vi "Main.vi"() -> ()   [LabVIEW 2010]
uses:
  <vilib>/Utility/config.llb/Read Key (Path).vi
  <vilib>/Utility/config.llb/Write Key (Path).vi
  DLL-s/MakeFullImmitationStepDLL/Release/MakeFullImmitationStepDLL.dll
  <vilib>/Utility/config.llb/NI_LVConfig.lvlib
panel:
  out "toChanger":T1(array[cluster])
  out "subpanel VI ref":refnum<vi>
  out "VP 2 GUI Msg Cluster Array":cluster{"Names":string[], "Codes":i32[]}
  out "selected path":path
  out "End Number":i32
  out "Project":string
  out "VP input vars":T2
  out "VP output vars":T3
  out "VM input vars":T2
  out "VM2SCM Msg Cluster Array":cluster{"Names":string[], "Codes":i32[]}
  out "VM INP from SCM Msg Cluster Array":cluster{"Names":string[], "Codes":i32[]}
  out "SCM2CA Msg Cluster Array":cluster{"Names":string[], "Codes":i32[]}
  out "SCM-SCM2VP Msg Cluster Array":cluster{"Names":string[], "Codes":i32[]}
  out "SCM2VM Msg Cluster Array":cluster{"Names":string[], "Codes":i32[]}
  out "VM2GUI Msg Cluster Array":cluster{"Names":string[], "Codes":i32[]}
  out "SCM STATES":string[][](array[string])
  out "SCM PROCESSES":string[](array[string])=["Инициализация", "ОстановВсехПроцессовИстартПроцИнициализация", "КонтрольДостоверности", "КонтрольДостоверностиОткрытияЗатвораВакуумного", "КонтрольДостоверностиОткрЗатВакуумного", "КонтрольДостоверностиЗакрЗатВакуумного", "КонтрольДостоверностиСостоянияСапуна", "КонтрольДостоверностиСостоянияУстройстваПлавПуска", "КонтрольДостоверностиСостоянияПитанияВакуумногоНасоса", "КонтрольДостоверностиСостоянияПитанияВентилятора", "КонтрольДостоверностиСостоянияПитанияРегТемпературы", "КонтрольДостоверностиСостоянияПитанияРегУровня", "КонтрольДостоверностиУровняВодыМинимум", "КонтрольДостоверностиУровняВодыМаксимум", "КонтрольДостоверностиСостоянияПитанияНасОхлаждения", "ЧтениеФактПараметров_с_Датчиков", "РЕГУЛЯТОР_ТРАФИКА", "ЧтениеКольцевогоБуфера", "ОбработкаКомандИзмененияНП_от_ГУИ", "ОбработкаКомандУправления_от_ГУИ", "КонтрольИзменения_ФП_P_ВбакеКомпрессора", "КонтрольИзменения_ФП_P_Впатрубке", "КонтрольИзменения_ФП_T_Врубашке", "КонтрольИзменения_ФП_T_Вбаке", "КонтрольИзменения_ФП_P_ВтрубеСидер", "КонтрольВеличиныОткачкиВауумнойТрубыСидеростата", "КонтрольГотовностиВакуума_в_Вакуумной_Трубе", "КонтрольУровняВодыБакаОхлаждения", "КонтрольТемпературыВодыБакаОхлаждения", "КонтрольТемпературыРубашкиОхлаждения", "КонтрольДавленияВбакеКомпрессора", "ВКЛ_ПИТ_ВЕНТИЛЯТОР", "ВЫК_ПИТ_ВЕНТИЛЯТОР", "КонтрольСостоянияПитанияВентилятора", "КонтрольСпонтанногоВыключенияВентилятора", "КонтрольСпонтанногоВключенияВентилятора", "КонтрольСостоянияЗатвораВакуумного", "ОТКР_ЗАТВОР_ВАК", "ЗАКР_ЗАТВОР_ВАК", "КонтрольСпонтанногоЗакрытияЗатвораВакуумного", "КонтрольСпонтанногоОткрытияЗатвораВакуумного", "ОТКР_САПУН", "ЗАКР_САПУН", "КонтрольСостоянияПитанияСапуна", "КонтрольСпонтанногоЗакрытияСапуна", "КонтрольСпонтанногоОткрытияСапуна", "ВКЛ_ПИТ_ВАК_НАСОСА", "ВЫК_ПИТ_ВАК_НАСОСА", "КонтрольСостоянияПитанияВакуумногоНасоса", "КонтрольСпонтанногоВыключенияВакНасоса", "КонтрольСпонтанногоВключенияВакНасоса", "ВКЛ_ПИТ_РЕГ_Т", "ВЫК_ПИТ_РЕГ_Т", "КонтрольСостоянияПитанияРЕГ_Т", "КонтрольСпонтанногоВыключенияРЕГ_Т", "КонтрольСпонтанногоВключенияРЕГ_Т", "ВКЛ_ПИТ_РЕГ_УР", "ВЫК_ПИТ_РЕГ_УР", "КонтрольСостоянияПитанияРЕГ_УР", "КонтрольСпонтанногоВыключенияРЕГ_УР", "КонтрольСпонтанногоВключенияРЕГ_УР", "ВКЛ_ПИТ_НАС_ОХЛ", "ВЫК_ПИТ_НАС_ОХЛ", "КонтрольСостоянияПитанияНАС_ОХЛ", "КонтрольСпонтанногоВыключенияНасосаОхлаждения", "КонтрольСпонтанногоВключенияНасосаОхлаждения", "ВКЛ_УСТР_ПЛАВ_ПУСКА", "ВЫК_УСТР_ПЛАВ_ПУСКА", "КонтрольСостоянияПитанияПЛАВ_ПУСКА", "КонтрольСпонтанногоВыключенияПлавнПуска", "КонтрольСпонтанногоВключенияПлавнПуска", "ВКЛ_ВАКУУМИРОВАНИЕ_ТРУБЫ", "ВЫК_ВАКУУМИРОВАНИЕ_ТРУБЫ", "ВКЛ_ВАКУУМНУЮ_ПОДСИСТЕМУ", "ВЫК_ВАКУУМНУЮ_ПОДСИСТЕМУ"]
  out "VM STATES":string[][](array[string])
  out "VM PROCESSES":string[](array[string])=["Инициализация", "ОстановВсехПроцессовИстартПроцИнициализация", "КонтрольДостоверности", "КонтрольДостоверностиОткрытияЗатвораВакуумного", "КонтрольДостоверностиОткрЗатВакуумного", "КонтрольДостоверностиЗакрЗатВакуумного", "КонтрольДостоверностиСостоянияСапуна", "КонтрольДостоверностиСостоянияУстройстваПлавПуска", "КонтрольДостоверностиСостоянияПитанияВакуумногоНасоса", "КонтрольДостоверностиСостоянияПитанияВентилятора", "КонтрольДостоверностиСостоянияПитанияРегТемпературы", "КонтрольДостоверностиСостоянияПитанияРегУровня", "КонтрольДостоверностиУровняВодыМинимум", "КонтрольДостоверностиУровняВодыМаксимум", "КонтрольДостоверностиСостоянияПитанияНасОхлаждения", "ЧтениеФактПараметров_с_Датчиков", "РЕГУЛЯТОР_ТРАФИКА", "ЧтениеКольцевогоБуфера", "ОбработкаКомандИзмененияНП_от_ГУИ", "ОбработкаКомандУправления_от_ГУИ", "КонтрольИзменения_ФП_P_ВбакеКомпрессора", "КонтрольИзменения_ФП_P_Впатрубке", "КонтрольИзменения_ФП_T_Врубашке", "КонтрольИзменения_ФП_T_Вбаке", "КонтрольИзменения_ФП_P_ВтрубеСидер", "КонтрольВеличиныОткачкиВауумнойТрубыСидеростата", "КонтрольГотовностиВакуума_в_Вакуумной_Трубе", "КонтрольУровняВодыБакаОхлаждения", "КонтрольТемпературыВодыБакаОхлаждения", "КонтрольТемпературыРубашкиОхлаждения", "КонтрольДавленияВбакеКомпрессора", "ВКЛ_ПИТ_ВЕНТИЛЯТОР", "ВЫК_ПИТ_ВЕНТИЛЯТОР", "КонтрольСостоянияПитанияВентилятора", "КонтрольСпонтанногоВыключенияВентилятора", "КонтрольСпонтанногоВключенияВентилятора", "КонтрольСостоянияЗатвораВакуумного", "ОТКР_ЗАТВОР_ВАК", "ЗАКР_ЗАТВОР_ВАК", "КонтрольСпонтанногоЗакрытияЗатвораВакуумного", "КонтрольСпонтанногоОткрытияЗатвораВакуумного", "ОТКР_САПУН", "ЗАКР_САПУН", "КонтрольСостоянияПитанияСапуна", "КонтрольСпонтанногоЗакрытияСапуна", "КонтрольСпонтанногоОткрытияСапуна", "ВКЛ_ПИТ_ВАК_НАСОСА", "ВЫК_ПИТ_ВАК_НАСОСА", "КонтрольСостоянияПитанияВакуумногоНасоса", "КонтрольСпонтанногоВыключенияВакНасоса", "КонтрольСпонтанногоВключенияВакНасоса", "ВКЛ_ПИТ_РЕГ_Т", "ВЫК_ПИТ_РЕГ_Т", "КонтрольСостоянияПитанияРЕГ_Т", "КонтрольСпонтанногоВыключенияРЕГ_Т", "КонтрольСпонтанногоВключенияРЕГ_Т", "ВКЛ_ПИТ_РЕГ_УР", "ВЫК_ПИТ_РЕГ_УР", "КонтрольСостоянияПитанияРЕГ_УР", "КонтрольСпонтанногоВыключенияРЕГ_УР", "КонтрольСпонтанногоВключенияРЕГ_УР", "ВКЛ_ПИТ_НАС_ОХЛ", "ВЫК_ПИТ_НАС_ОХЛ", "КонтрольСостоянияПитанияНАС_ОХЛ", "КонтрольСпонтанногоВыключенияНасосаОхлаждения", "КонтрольСпонтанногоВключенияНасосаОхлаждения", "ВКЛ_УСТР_ПЛАВ_ПУСКА", "ВЫК_УСТР_ПЛАВ_ПУСКА", "КонтрольСостоянияПитанияПЛАВ_ПУСКА", "КонтрольСпонтанногоВыключенияПлавнПуска", "КонтрольСпонтанногоВключенияПлавнПуска", "ВКЛ_ВАКУУМИРОВАНИЕ_ТРУБЫ", "ВЫК_ВАКУУМИРОВАНИЕ_ТРУБЫ", "ВКЛ_ВАКУУМНУЮ_ПОДСИСТЕМУ", "ВЫК_ВАКУУМНУЮ_ПОДСИСТЕМУ"]
  out "VP STATES":string[][](array[string])
  out "VP PROCESSES":string[](array[string])=["Инициализация", "ОстановВсехПроцессовИстартПроцИнициализация", "КонтрольДостоверности", "КонтрольДостоверностиОткрытияЗатвораВакуумного", "КонтрольДостоверностиОткрЗатВакуумного", "КонтрольДостоверностиЗакрЗатВакуумного", "КонтрольДостоверностиСостоянияСапуна", "КонтрольДостоверностиСостоянияУстройстваПлавПуска", "КонтрольДостоверностиСостоянияПитанияВакуумногоНасоса", "КонтрольДостоверностиСостоянияПитанияВентилятора", "КонтрольДостоверностиСостоянияПитанияРегТемпературы", "КонтрольДостоверностиСостоянияПитанияРегУровня", "КонтрольДостоверностиУровняВодыМинимум", "КонтрольДостоверностиУровняВодыМаксимум", "КонтрольДостоверностиСостоянияПитанияНасОхлаждения", "ЧтениеФактПараметров_с_Датчиков", "РЕГУЛЯТОР_ТРАФИКА", "ЧтениеКольцевогоБуфера", "ОбработкаКомандИзмененияНП_от_ГУИ", "ОбработкаКомандУправления_от_ГУИ", "КонтрольИзменения_ФП_P_ВбакеКомпрессора", "КонтрольИзменения_ФП_P_Впатрубке", "КонтрольИзменения_ФП_T_Врубашке", "КонтрольИзменения_ФП_T_Вбаке", "КонтрольИзменения_ФП_P_ВтрубеСидер", "КонтрольВеличиныОткачкиВауумнойТрубыСидеростата", "КонтрольГотовностиВакуума_в_Вакуумной_Трубе", "КонтрольУровняВодыБакаОхлаждения", "КонтрольТемпературыВодыБакаОхлаждения", "КонтрольТемпературыРубашкиОхлаждения", "КонтрольДавленияВбакеКомпрессора", "ВКЛ_ПИТ_ВЕНТИЛЯТОР", "ВЫК_ПИТ_ВЕНТИЛЯТОР", "КонтрольСостоянияПитанияВентилятора", "КонтрольСпонтанногоВыключенияВентилятора", "КонтрольСпонтанногоВключенияВентилятора", "КонтрольСостоянияЗатвораВакуумного", "ОТКР_ЗАТВОР_ВАК", "ЗАКР_ЗАТВОР_ВАК", "КонтрольСпонтанногоЗакрытияЗатвораВакуумного", "КонтрольСпонтанногоОткрытияЗатвораВакуумного", "ОТКР_САПУН", "ЗАКР_САПУН", "КонтрольСостоянияПитанияСапуна", "КонтрольСпонтанногоЗакрытияСапуна", "КонтрольСпонтанногоОткрытияСапуна", "ВКЛ_ПИТ_ВАК_НАСОСА", "ВЫК_ПИТ_ВАК_НАСОСА", "КонтрольСостоянияПитанияВакуумногоНасоса", "КонтрольСпонтанногоВыключенияВакНасоса", "КонтрольСпонтанногоВключенияВакНасоса", "ВКЛ_ПИТ_РЕГ_Т", "ВЫК_ПИТ_РЕГ_Т", "КонтрольСостоянияПитанияРЕГ_Т", "КонтрольСпонтанногоВыключенияРЕГ_Т", "КонтрольСпонтанногоВключенияРЕГ_Т", "ВКЛ_ПИТ_РЕГ_УР", "ВЫК_ПИТ_РЕГ_УР", "КонтрольСостоянияПитанияРЕГ_УР", "КонтрольСпонтанногоВыключенияРЕГ_УР", "КонтрольСпонтанногоВключенияРЕГ_УР", "ВКЛ_ПИТ_НАС_ОХЛ", "ВЫК_ПИТ_НАС_ОХЛ", "КонтрольСостоянияПитанияНАС_ОХЛ", "КонтрольСпонтанногоВыключенияНасосаОхлаждения", "КонтрольСпонтанногоВключенияНасосаОхлаждения", "ВКЛ_УСТР_ПЛАВ_ПУСКА", "ВЫК_УСТР_ПЛАВ_ПУСКА", "КонтрольСостоянияПитанияПЛАВ_ПУСКА", "КонтрольСпонтанногоВыключенияПлавнПуска", "КонтрольСпонтанногоВключенияПлавнПуска", "ВКЛ_ВАКУУМИРОВАНИЕ_ТРУБЫ", "ВЫК_ВАКУУМИРОВАНИЕ_ТРУБЫ", "ВКЛ_ВАКУУМНУЮ_ПОДСИСТЕМУ", "ВЫК_ВАКУУМНУЮ_ПОДСИСТЕМУ"]
  out "VP Cluster":T4
  out "CA output vars":T3
  out "CA input vars":T2
  out "CA2GUI Msg Cluster Array":cluster{"Names":string[], "Codes":i32[]}
  out "COM2CA MSG Cluster Array":cluster{"Names":string[], "Codes":i32[]}
  out "CA STATES":string[][](array[string])
  out "CA PROCESSES":string[](array[string])=["Инициализация", "ОстановВсехПроцессовИстартПроцИнициализация", "КонтрольДостоверности", "КонтрольДостоверностиОткрытияЗатвораВакуумного", "КонтрольДостоверностиОткрЗатВакуумного", "КонтрольДостоверностиЗакрЗатВакуумного", "КонтрольДостоверностиСостоянияСапуна", "КонтрольДостоверностиСостоянияУстройстваПлавПуска", "КонтрольДостоверностиСостоянияПитанияВакуумногоНасоса", "КонтрольДостоверностиСостоянияПитанияВентилятора", "КонтрольДостоверностиСостоянияПитанияРегТемпературы", "КонтрольДостоверностиСостоянияПитанияРегУровня", "КонтрольДостоверностиУровняВодыМинимум", "КонтрольДостоверностиУровняВодыМаксимум", "КонтрольДостоверностиСостоянияПитанияНасОхлаждения", "ЧтениеФактПараметров_с_Датчиков", "РЕГУЛЯТОР_ТРАФИКА", "ЧтениеКольцевогоБуфера", "ОбработкаКомандИзмененияНП_от_ГУИ", "ОбработкаКомандУправления_от_ГУИ", "КонтрольИзменения_ФП_P_ВбакеКомпрессора", "КонтрольИзменения_ФП_P_Впатрубке", "КонтрольИзменения_ФП_T_Врубашке", "КонтрольИзменения_ФП_T_Вбаке", "КонтрольИзменения_ФП_P_ВтрубеСидер", "КонтрольВеличиныОткачкиВауумнойТрубыСидеростата", "КонтрольГотовностиВакуума_в_Вакуумной_Трубе", "КонтрольУровняВодыБакаОхлаждения", "КонтрольТемпературыВодыБакаОхлаждения", "КонтрольТемпературыРубашкиОхлаждения", "КонтрольДавленияВбакеКомпрессора", "ВКЛ_ПИТ_ВЕНТИЛЯТОР", "ВЫК_ПИТ_ВЕНТИЛЯТОР", "КонтрольСостоянияПитанияВентилятора", "КонтрольСпонтанногоВыключенияВентилятора", "КонтрольСпонтанногоВключенияВентилятора", "КонтрольСостоянияЗатвораВакуумного", "ОТКР_ЗАТВОР_ВАК", "ЗАКР_ЗАТВОР_ВАК", "КонтрольСпонтанногоЗакрытияЗатвораВакуумного", "КонтрольСпонтанногоОткрытияЗатвораВакуумного", "ОТКР_САПУН", "ЗАКР_САПУН", "КонтрольСостоянияПитанияСапуна", "КонтрольСпонтанногоЗакрытияСапуна", "КонтрольСпонтанногоОткрытияСапуна", "ВКЛ_ПИТ_ВАК_НАСОСА", "ВЫК_ПИТ_ВАК_НАСОСА", "КонтрольСостоянияПитанияВакуумногоНасоса", "КонтрольСпонтанногоВыключенияВакНасоса", "КонтрольСпонтанногоВключенияВакНасоса", "ВКЛ_ПИТ_РЕГ_Т", "ВЫК_ПИТ_РЕГ_Т", "КонтрольСостоянияПитанияРЕГ_Т", "КонтрольСпонтанногоВыключенияРЕГ_Т", "КонтрольСпонтанногоВключенияРЕГ_Т", "ВКЛ_ПИТ_РЕГ_УР", "ВЫК_ПИТ_РЕГ_УР", "КонтрольСостоянияПитанияРЕГ_УР", "КонтрольСпонтанногоВыключенияРЕГ_УР", "КонтрольСпонтанногоВключенияРЕГ_УР", "ВКЛ_ПИТ_НАС_ОХЛ", "ВЫК_ПИТ_НАС_ОХЛ", "КонтрольСостоянияПитанияНАС_ОХЛ", "КонтрольСпонтанногоВыключенияНасосаОхлаждения", "КонтрольСпонтанногоВключенияНасосаОхлаждения", "ВКЛ_УСТР_ПЛАВ_ПУСКА", "ВЫК_УСТР_ПЛАВ_ПУСКА", "КонтрольСостоянияПитанияПЛАВ_ПУСКА", "КонтрольСпонтанногоВыключенияПлавнПуска", "КонтрольСпонтанногоВключенияПлавнПуска", "ВКЛ_ВАКУУМИРОВАНИЕ_ТРУБЫ", "ВЫК_ВАКУУМИРОВАНИЕ_ТРУБЫ", "ВКЛ_ВАКУУМНУЮ_ПОДСИСТЕМУ", "ВЫК_ВАКУУМНУЮ_ПОДСИСТЕМУ"]
  out "CA DESCR":T5
  out "VM DESCR":T6
  out "exists":bool
  out "Scalar":bool
  in  "Проект":path
  out "Stop Ver Button":bool
  in  "Pause":bool
  out "Верификация запущена":bool
  out "error":i32
  in  "verifier2scenariousControlOutMsgs":cluster{"MSG":i16, "param":i32, "Type":i16}[](array[cluster])
  out "Verification":bool
  in  "scenarioStates":cluster{"TimeInState":u16, "cur_state":i8}[](array[cluster])
  in  "verStates":cluster{"TimeInState":u16, "cur_state":i8}[](array[cluster])
  in  "vplantStates":cluster{"TimeInState":u16, "cur_state":i8}[](array[cluster])
  in  "algStates":cluster{"TimeInState":u16, "cur_state":i8}[](array[cluster])
  in  "virtualPlant2GUIOutputMsgs":cluster{"MSG":i16, "param":i32, "Type":i16}[](array[cluster])
  in  "verifier2GUIOutputMsgs":cluster{"MSG":i16, "param":i32, "Type":i16}[](array[cluster])
  in  "algOutputMsgs":T7(array[cluster])
  in  "scenarios2VerifierOutputMsgs":cluster{"MSG":i16, "param":i32, "Type":i16}[](array[cluster])
  in  "scenarios2VirtPlantOutputMsgs":cluster{"MSG":i16, "param":i32, "Type":i16}[](array[cluster])
  in  "scenarios2AlgOutputMsgs":cluster{"MSG":i16, "param":i32, "Type":i16}[](array[cluster])
  in  "algOutputPorts":i8[](array[numeric])
  in  "algInputPorts":i8[](array[numeric])
  in  "TEST MODE":bool
  in  "Open editor":bool
  in  "START Button":bool
  out "VM vi reference":refnum<vi> caption="CA vi reference"
  out "SCB vi reference":refnum<vi> caption="CA vi reference"
  out "VP vi reference":refnum<vi> caption="CA vi reference"
  out "CA vi reference":refnum<vi>
  out "error out":errorcluster
  in  "Открыть панель БВ":bool
  in  "Открыть панель БУС":bool
  in  "Открыть панель АУ":bool
  in  "stop":bool
  in  "Открыть панель ВОУ":bool
  out "Автоматический режим работы":bool
  in  "Режим работы:":bool
  # "Ручной"
  # "Автоматический"
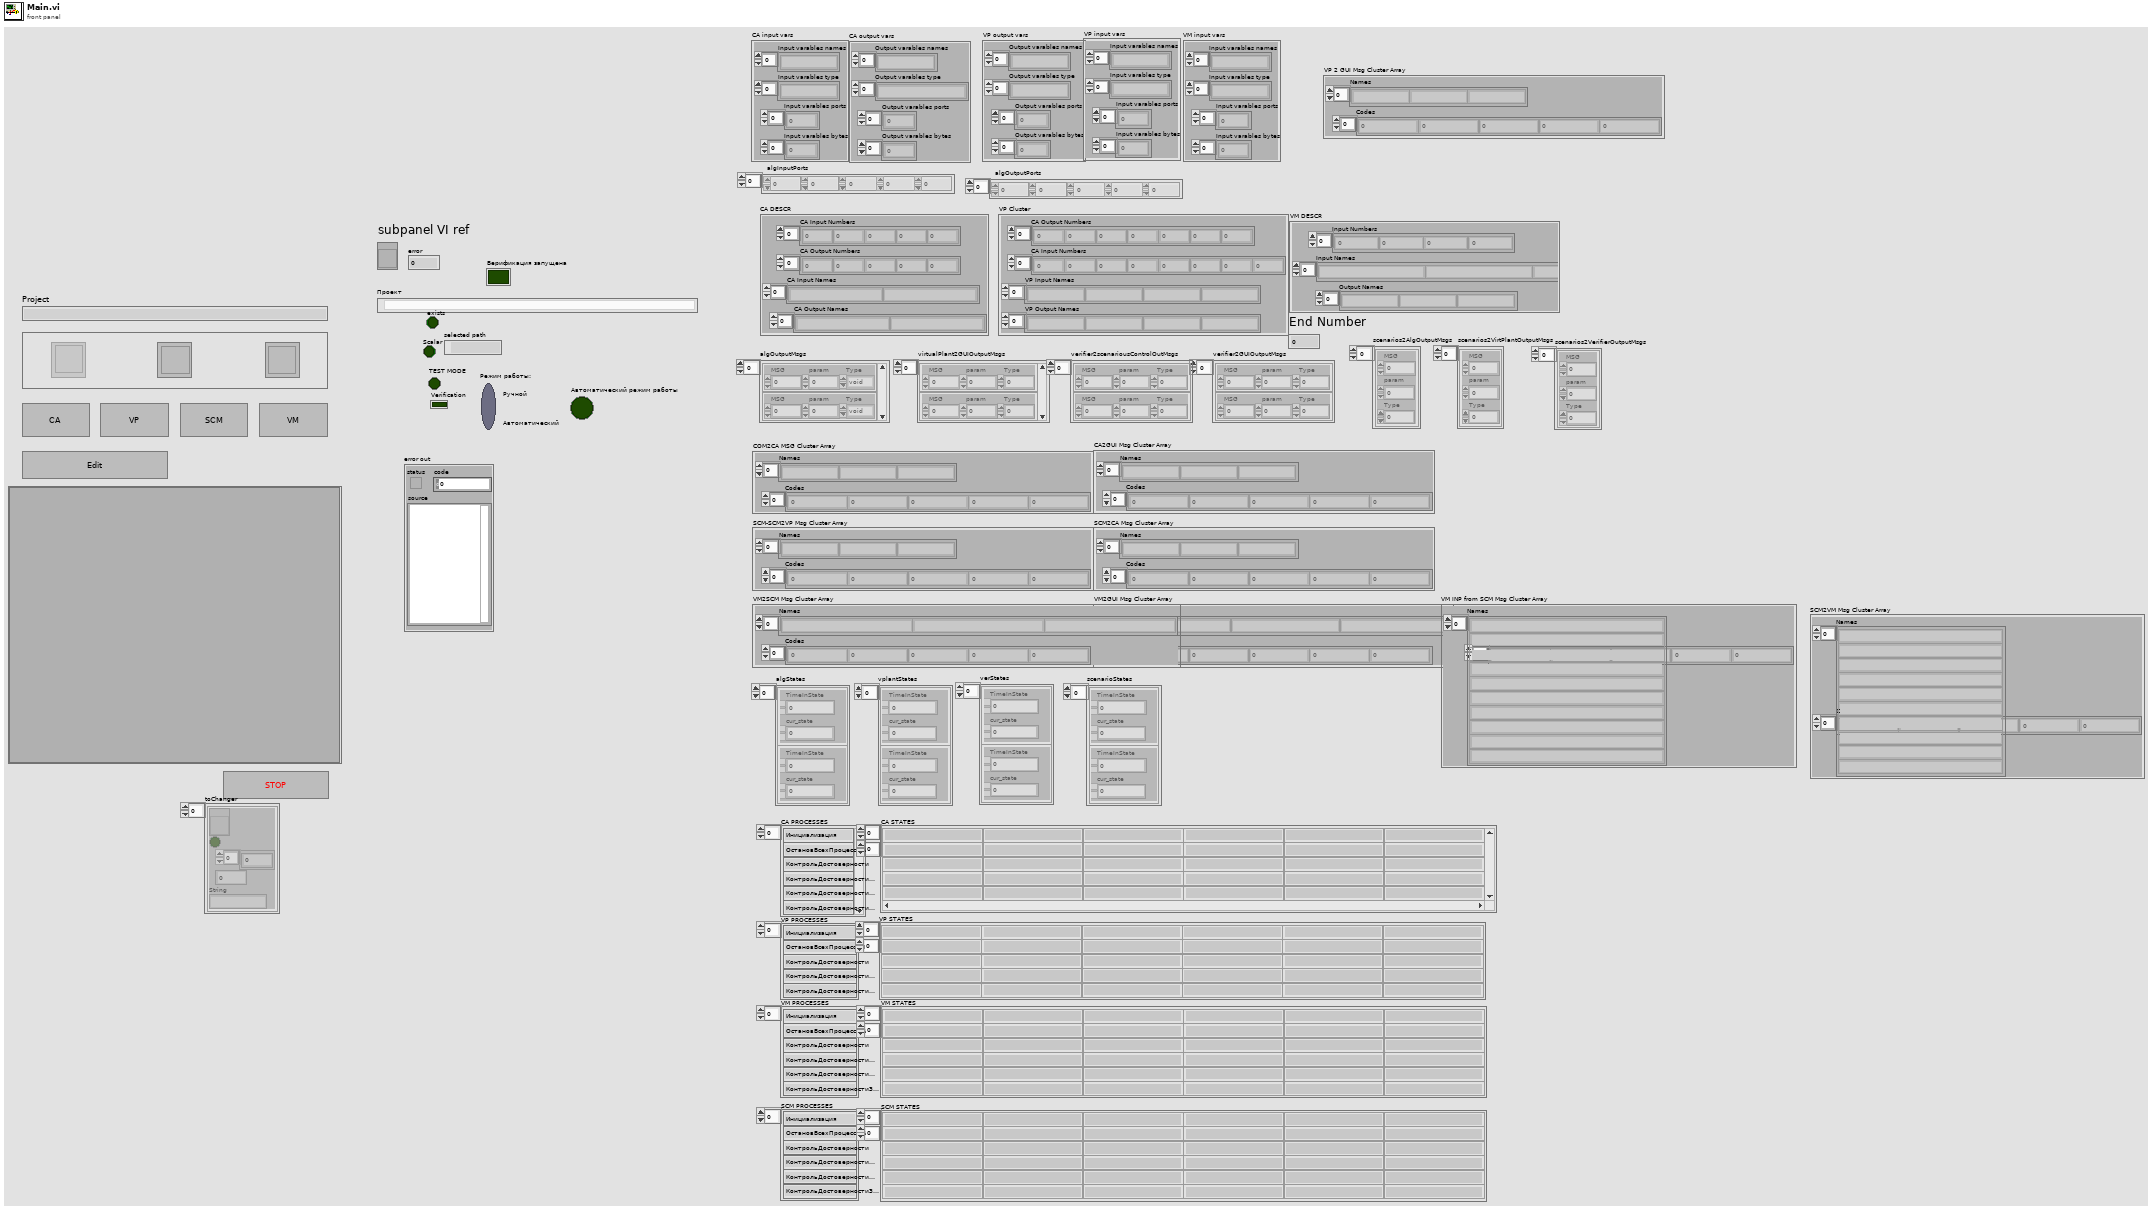
[diagram p1: front panel]
types:
  T1 = cluster{refnum<vi>, bool, i32[], i32, "String":string}[]
  T2 = cluster{"Input varables names":string[], "Input varables type":string[], "Input varables ports":i32[], "Input varables bytes":i32[]}
  T3 = cluster{"Output varables names":string[], "Output varables type":string[], "Output varables ports":i32[], "Output varables bytes":i32[]}
  T4 = cluster{"CA Output Numbers ":i32[], "CA Input Numbers":i32[], "VP Input Names":string[], "VP Output Names ":string[]}
  T5 = cluster{"CA Input Numbers":i32[], "CA Output Numbers ":i32[], "CA Input Names":string[], "CA Output Names ":string[]}
  T6 = cluster{"Input Numbers":i32[], "Input Names":string[], "Output Names ":string[]}
  T7 = cluster{"MSG":i16, "param":i32, "Type":enum16{"void", "byte", "int", "float"}}[]
  T8 = enum8{"Enabled", "Disabled", "Disabled and Grayed Out"}
  T9 = typedef "NI_LVConfig.lvlib/Config Data RefNum.ctl" = refnum<k1>
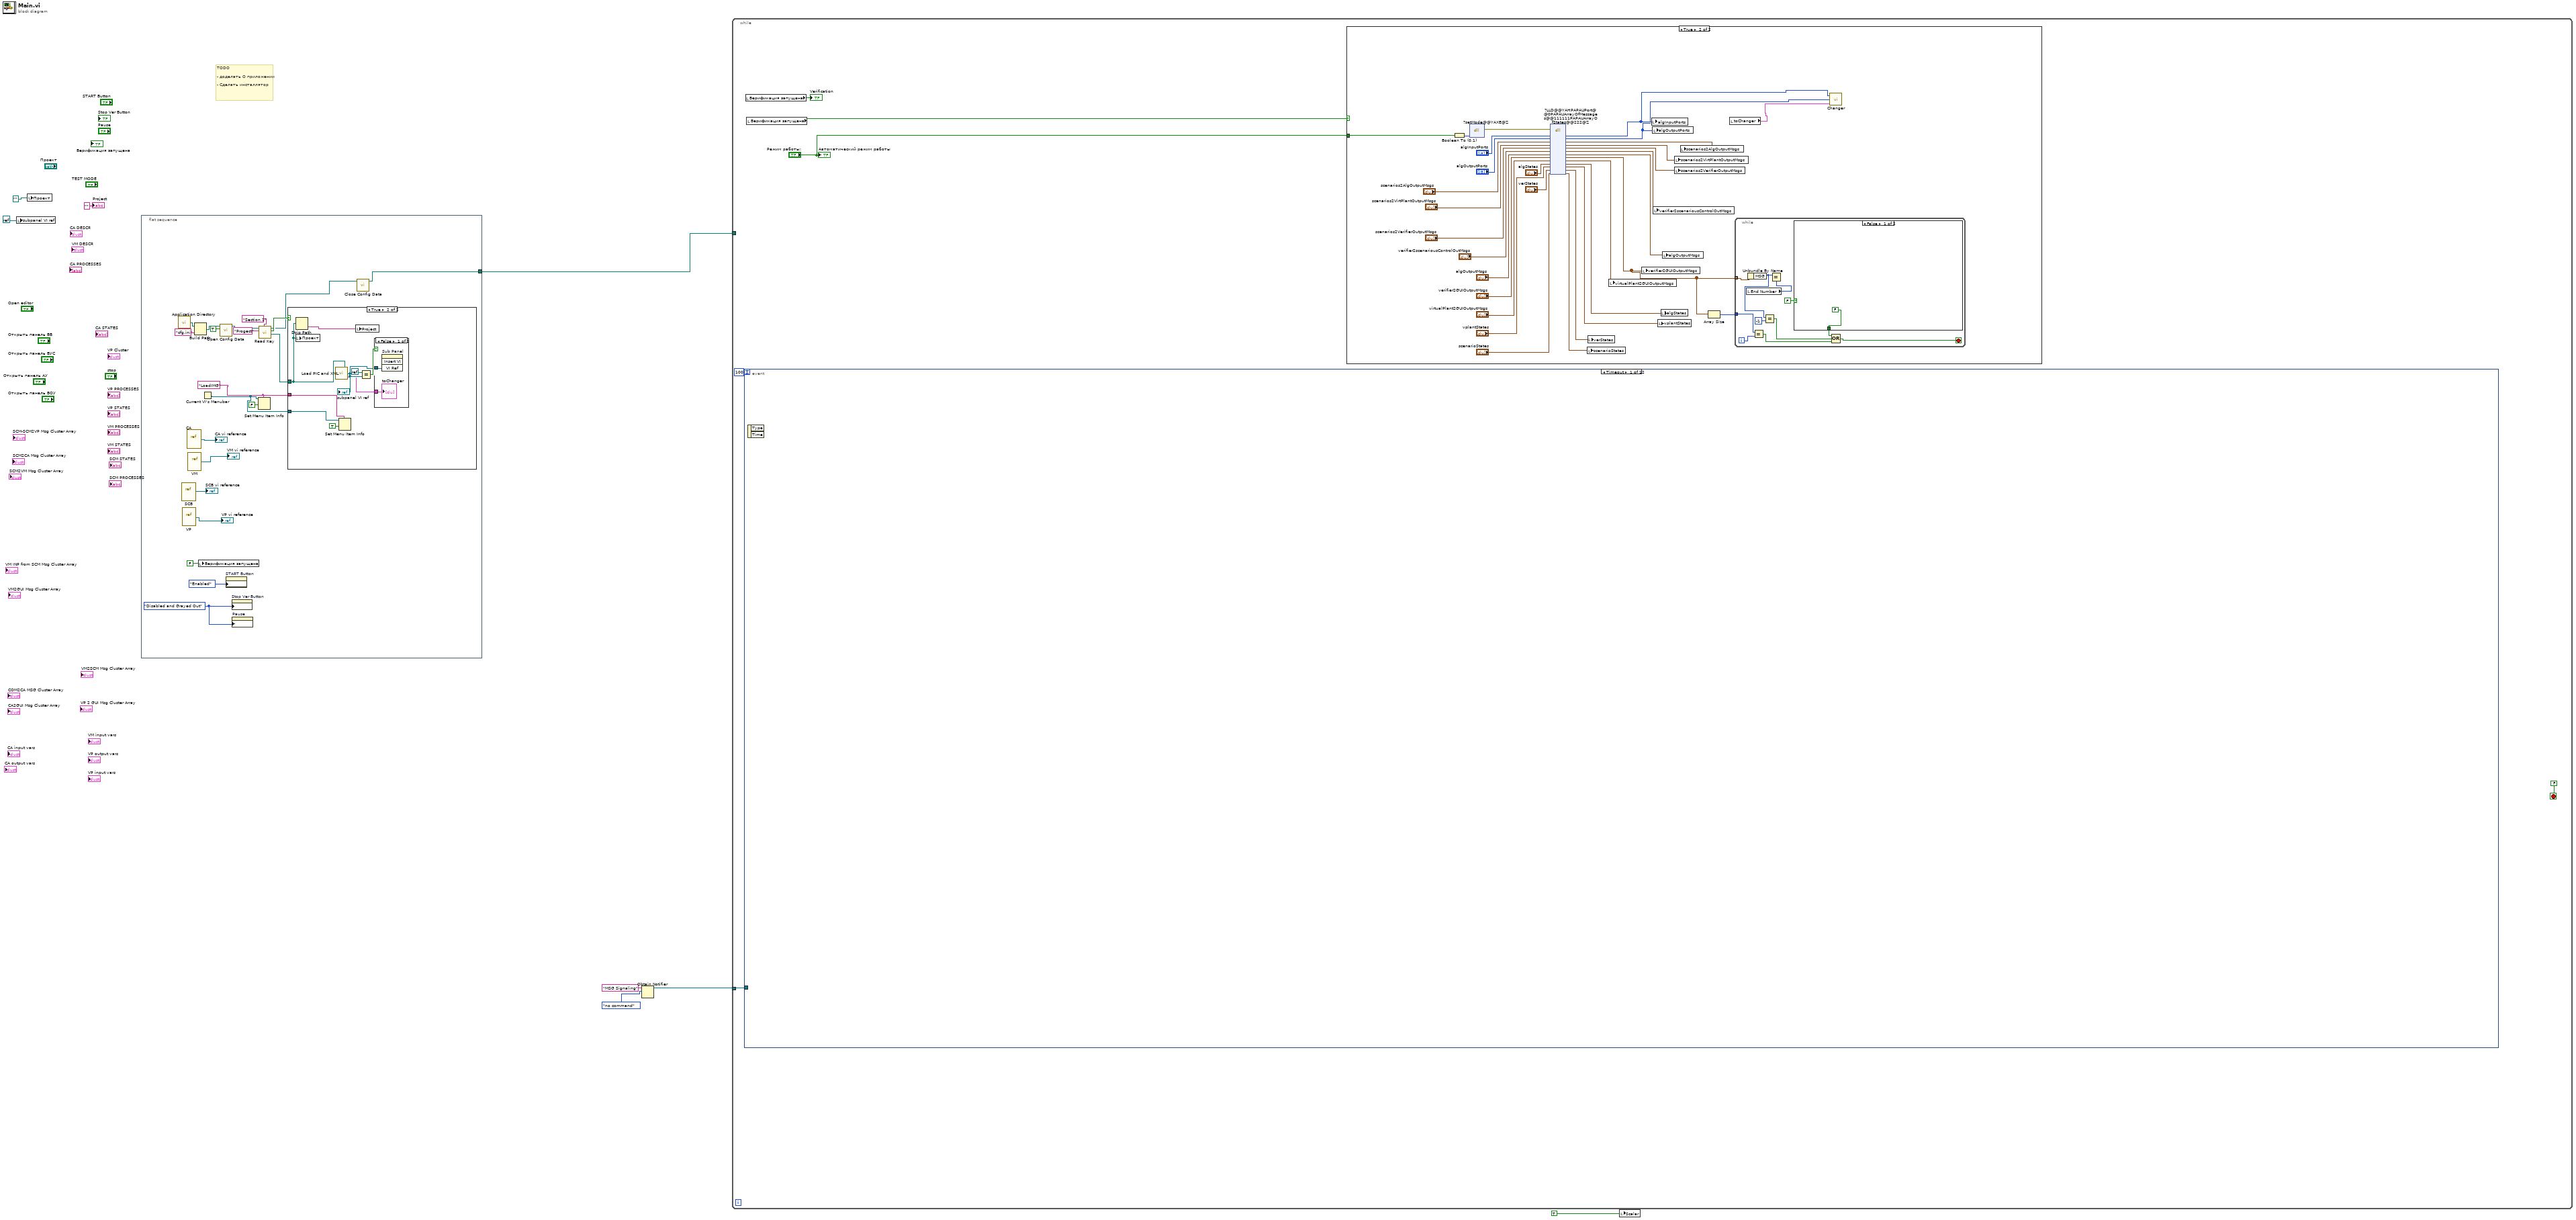
[diagram p0: block diagram]
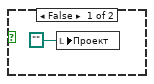
[diagram p2: hidden frame]
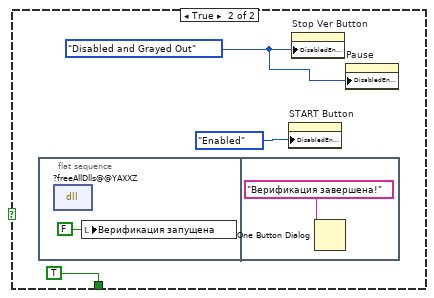
[diagram p5: hidden frame]
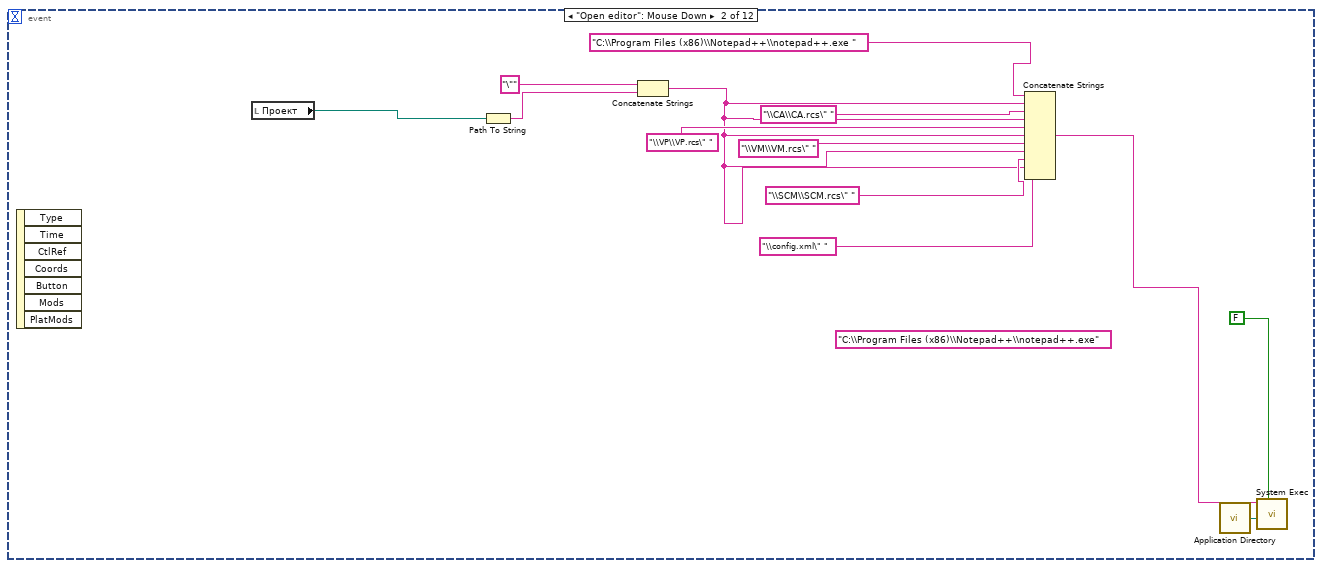
[diagram p6: hidden frame]
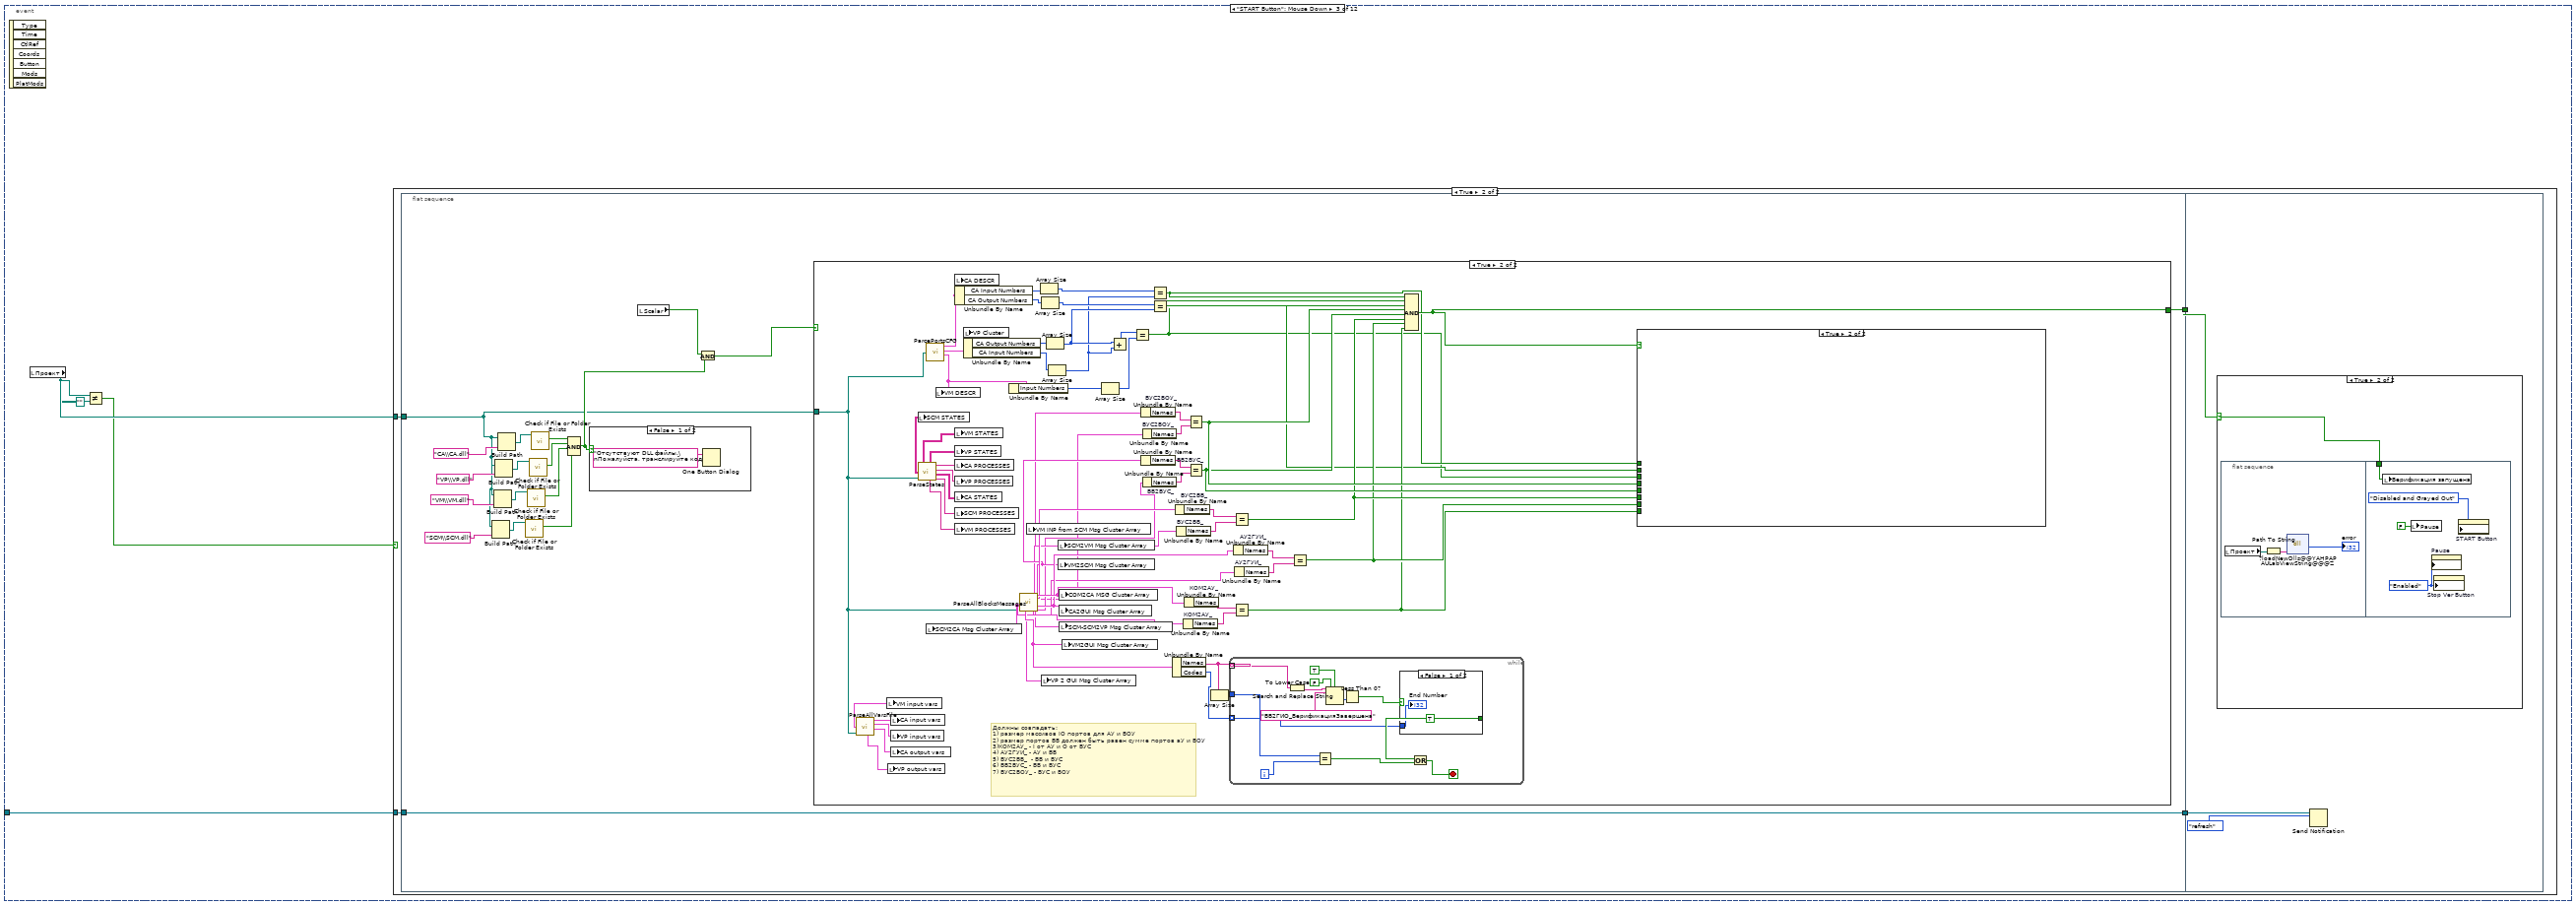
[diagram p7: hidden frame]
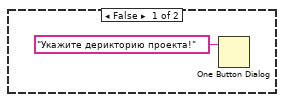
[diagram p8: hidden frame]
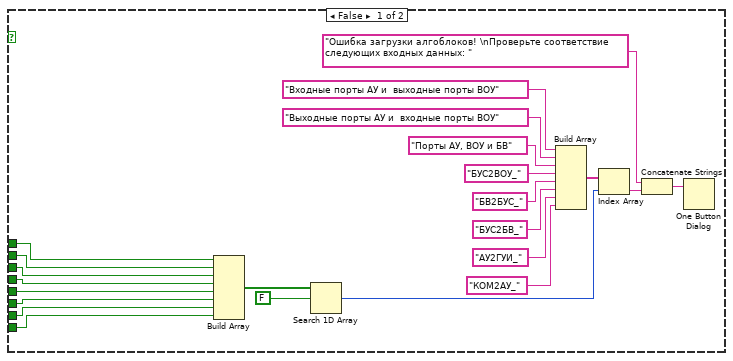
[diagram p11: hidden frame]
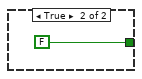
[diagram p12: hidden frame]
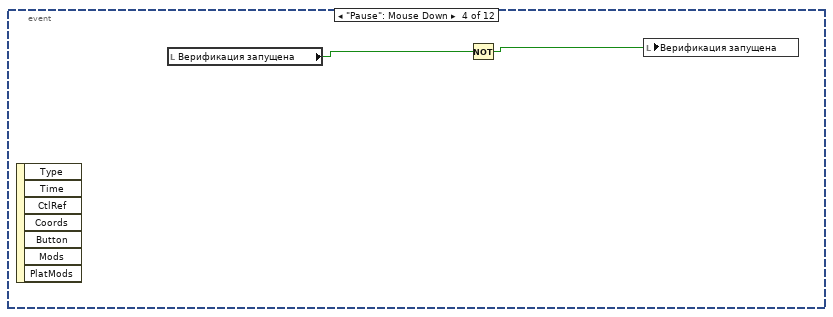
[diagram p14: hidden frame]
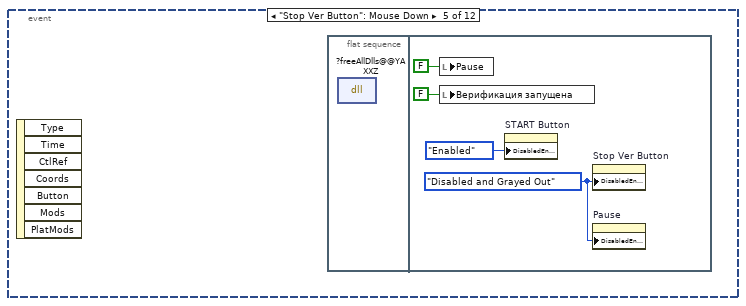
[diagram p15: hidden frame]
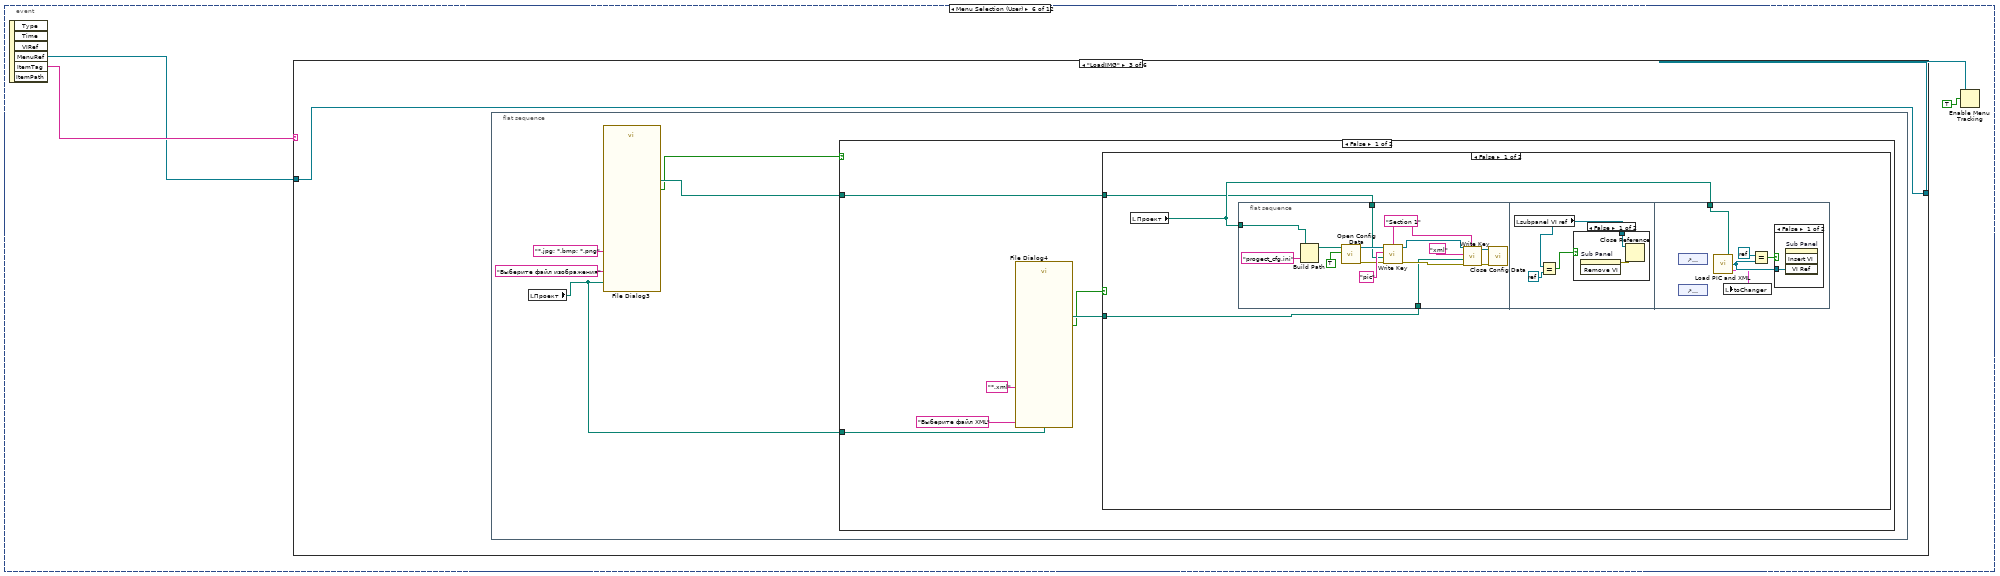
[diagram p16: hidden frame]
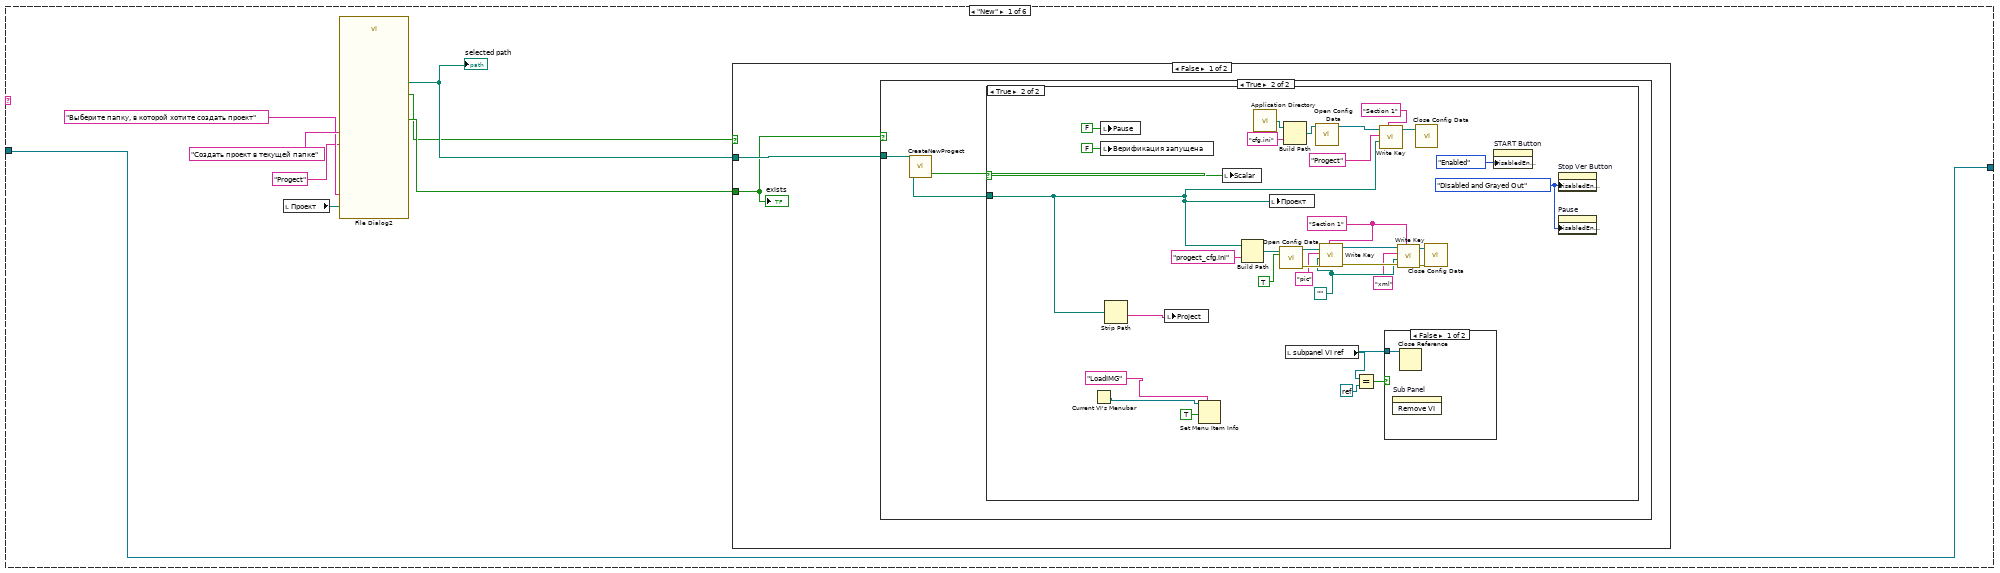
[diagram p17: hidden frame]
diagram:
  # "TODO\n\n- доделать О приложении\n\n- Сделать инсталлятор"
  n1 = local write "subpanel VI ref"(refnum<k0> refnum) -> ()
  n2 = local write "Проект"(path "") -> ()
  n3 = flat-sequence {
    tunnel: [w16] -> w3
    frame #0 {
      w14 = "LoadIMG" ("item tag")
      w27 = T8."Disabled and Grayed Out" ("Disabled")
      n4 = call <vilib>:"Application Directory.vi"() -> ("Application Directory"=w26:path)
      n5 = vi-ref "SCB.vi"() -> (→"SCB vi reference":refnum<vi>)
      n6 = vi-ref "VP.vi"() -> (→"VP vi reference":refnum<vi>)
      n7 = vi-ref "CA.vi"() -> (→"CA vi reference":refnum<vi>)
      n8 = vi-ref "VM.vi"() -> (→"VM vi reference":refnum<vi>)
      n9 = Build Path(base path=w26, name or relative path="cfg.ini") -> (appended path=w24:path)
      n10 = local write "Верификация запущена"(FALSE ("VerificationRunning")) -> ()
      n11 = Current VI's Menubar() -> (w13:refnum<k9>)
      n12 = call <vilib>:"Open Config Data.vi"("create file if necessary (T)"=TRUE, "configuration file path"=w24) -> ("refnum"=w19:T9)  [unwired: 7 in, 2 out]
      n13 = property on="START Button" class="Bool (strict)"("DisabledEnum"=T8."Enabled" ("Disabled")) -> ()  [unwired: 2 in, 2 out]
      n14 = property on="Stop Ver Button" class="Bool (strict)"("DisabledEnum"=w27) -> ()  [unwired: 2 in, 2 out]
      n15 = property on="Pause" class="Bool (strict)"("DisabledEnum"=w27) -> ()  [unwired: 2 in, 2 out]
      n16 = Set Menu Item Info(7:w14, 9:FALSE ("enabled"), 11:w13) -> ()  [unwired: 4 in, 2 out]
      n17 = call-poly <vilib>:"Read Key.vi"("section"="Section 1", "key"="Progect", "refnum"=w19) -> ("value"=w20:path, "found?"=w21:bool, "refnum out"=w17:T9)  [unwired: 5 in, 1 out]
      n18 = case shown="True" w21 {
        tunnel: w20 -> [_ w39]
        tunnel: w14 -> [_ w33]
        tunnel: w13 -> [_ w32]
        frame False {
          n19 = local write "Проект"(path "") -> ()
        }
        frame True {
          n20 = Strip Path(path=w39) -> (name=w35:string)  [unwired: 1 out]
          n21 = local write "Проект"(w39) -> ()
          n22 = call "Load PIC and XML.vi"("selected path"=w39) -> ("toChanger"=w31:T1, "vi refnum"=w36:refnum<vi>)  [unwired: 2 in]
          "subpanel VI ref" <- w36
          n23 = Set Menu Item Info(7:w33, 9:TRUE ("enabled"), 11:w32) -> ()  [unwired: 4 in, 2 out]
          n24 = local write "Project"(w35) -> ()
          n25 = Equal?(x=refnum<k0> refnum, y=w36) -> (x = y?=w37:bool)
          n26 = case shown="False" w37 {
            tunnel: w36 -> [w41 _]
            tunnel: w31 -> [w40 _]
            frame False {
              n27 = invoke on="Sub Panel" class="SubPnl" method="Insert VI"("VI Ref"=w41) -> ()  [unwired: 3 in, 4 out]
              "toChanger" <- w40
            }
            frame True {
            }
          }
        }
      }
      n28 = call <vilib>:"Close Config Data.vi"("refnum"=w17) -> ("file path"=w16:path)  [unwired: 9 in, 1 out]
    }
  }
  n29 = Obtain Notifier(name (unnamed)="MSG Signaling", notification data type=enum16{"no command", "refresh"}."no command") -> (notifier out=w6:refnum<notifier>)  [unwired: 2 in, 2 out]
  n30 = while {
    tunnel: w6 -> [w43]
    tunnel: w3 -> [_]
    stop <- FALSE ("stop") stop-if-true
    n31 = event shown="[0] Timeout" {
      selector: _ -> [_ _ _ _ _ _ _ _ _ _ _ _]
      dyn-events: _ -> [_ _ _ _ _ _ _ _ _ _ _ _]
      timeout: 100 -> [_ _ _ _ _ _ _ _ _ _ _ _]
      tunnel: w43 -> [_ _ w112 _ _ _ _ _ _ _ _ _]
      event Timeout {
        n32 = event-data() -> ()  [unwired: 1 in, 2 out]
      }
      event "Open editor": Mouse Down {
        (unwired) "C:\\Program Files (x86)\\Notepad++\\notepad++.exe" ("command line")
        n33 = event-data() -> ()  [unwired: 1 in, 7 out]
        n34 = local read "Проект"() -> (w101:path)
        n35 = Path To String(path=w101) -> (string=w103:string)
        n36 = Concatenate Strings("\"" ("string"), w103) -> (w97:string)
        n37 = Concatenate Strings("C:\\Program Files (x86)\\Notepad++\\notepad++.exe " ("command line"), w97, "\\CA\\CA.rcs\" " ("string"), w97, "\\VP\\VP.rcs\" " ("string"), w97, "\\VM\\VM.rcs\" " ("string"), w97, "\\SCM\\SCM.rcs\" " ("string"), w97, "\\config.xml\" " ("string")) -> (w98:string)
        n38 = call <vilib>:"Application Directory.vi"() -> ("Application Directory"=w107:path)
        n39 = call <vilib>:"System Exec.vi"("wait until completion? (T)"=FALSE, "working directory"=w107, "command line"=w98) -> ()  [unwired: 5 in, 4 out]
      }
      event "START Button": Mouse Down {
        n40 = event-data() -> ()  [unwired: 1 in, 7 out]
        n41 = local read "Проект"() -> (w111:path)
        n42 = Not Equal?(x=w111, y=path "") -> (x != y?=w109:bool)
        n43 = case shown="True" w109 {
          tunnel: w112 -> [_ w115]
          tunnel: w111 -> [_ w114]
          frame False {
            n44 = One Button Dialog(message="Укажите дерикторию проекта!") -> ()  [unwired: 1 in, 1 out]
          }
          frame True {
            n45 = flat-sequence {
              tunnel: w115 -> [w135]
              tunnel: [w135] -> w117
              tunnel: [w134] -> w116
              tunnel: w114 -> [w118]
              tunnel: w117 -> [w241]
              tunnel: w116 -> [w239]
              frame #0 {
                n46 = Build Path(base path=w118, name or relative path="SCM\\SCM.dll") -> (appended path=w128:path)
                n47 = Build Path(base path=w118, name or relative path="VM\\VM.dll") -> (appended path=w129:path)
                n48 = Build Path(base path=w118, name or relative path="VP\\VP.dll") -> (appended path=w130:path)
                n49 = Build Path(base path=w118, name or relative path="CA\\CA.dll") -> (appended path=w132:path)
                n50 = call <vilib>:"Check if File or Folder Exists.vi"("path"=w128) -> ("file or folder exists?"=w119:bool)  [unwired: 8 in, 2 out]
                n51 = call <vilib>:"Check if File or Folder Exists.vi"("path"=w129) -> ("file or folder exists?"=w123:bool)  [unwired: 8 in, 2 out]
                n52 = call <vilib>:"Check if File or Folder Exists.vi"("path"=w130) -> ("file or folder exists?"=w124:bool)  [unwired: 8 in, 2 out]
                n53 = call <vilib>:"Check if File or Folder Exists.vi"("path"=w132) -> ("file or folder exists?"=w131:bool)  [unwired: 8 in, 2 out]
                n54 = Compound Arithmetic op=AND(w131, w124, w123, w119) -> (w122:bool)
                n55 = case shown="False" w122 {
                  frame False {
                    n56 = One Button Dialog(message="Отсутствуют DLL файлы.\nПожалуйста, транслируйте код.") -> ()  [unwired: 1 in, 1 out]
                  }
                  frame True {
                  }
                }
                n57 = local read "Scalar"() -> (w121:bool)
                n58 = And(x=w121, y=w122) -> (x .and. y?=w120:bool)
                n59 = case shown="True" w120 {
                  selector: w120 -> [w137 _]
                  tunnel: [w137 w143] -> w134
                  tunnel: w118 -> [_ w139]
                  frame False {
                  }
                  frame True {
                    # "Должны совпадать:\n1) размер массивов IO портов для АУ и ВОУ\n2) размер портов БВ должен быть равен сумме портов аУ и ВОУ\n3)КОМ2АУ_ - I от АУ и O от БУС\n4) АУ2ГУИ_ - АУ и БВ\n5) БУС2БВ_  - БВ и БУС\n6) БВ2БУС_ - БВ и БУС\n7) БУС2ВОУ_ - БУС и ВОУ"
                    n60 = call "ParseAllVarsFile.vi"("Path"=w139) -> ("CA input vars"=w197:T2, "VP input vars"=w187:T2, "CA output vars"=w196:T3, "VP output vars"=w188:T3, "VM input vars"=w189:T2)  [unwired: 3 out]
                    n61 = local write "VM input vars"(w189) -> ()
                    n62 = local write "VP output vars"(w188) -> ()
                    n63 = local write "CA input vars"(w197) -> ()
                    n64 = local write "VP input vars"(w187) -> ()
                    n65 = local write "CA output vars"(w196) -> ()
                    n66 = call "ParseStates.vi"("base path"=w139) -> ("CA PROCESSES"=w199:string[], "VP STATES"=w194:string[][], "VP PROCESSES"=w195:string[], "CA STATES"=w198:string[][], "VM PROCESSES"=w193:string[], "SCM PROCESSES"=w191:string[], "VM STATES"=w192:string[][], "SCM STATES"=w190:string[][])
                    n67 = local write "SCM STATES"(w190) -> ()
                    n68 = call "ParcePortsCFG.vi"("path"=w139) -> ("VM Cluster"=w175:T6, "VP Cluster"=w182:T4, "CA Cluster"=w183:T5)  [unwired: 1 out]
                    n69 = local write "VM DESCR"(w175) -> ()
                    n70 = local write "CA DESCR"(w183) -> ()
                    n71 = Unbundle By Name(w183) -> ("CA Input Numbers"=w181:i32[], "CA Output Numbers"=w180:i32[])
                    n72 = local write "VM STATES"(w192) -> ()
                    n73 = local write "VP STATES"(w194) -> ()
                    n74 = local write "CA PROCESSES"(w199) -> ()
                    n75 = local write "VP PROCESSES"(w195) -> ()
                    n76 = local write "CA STATES"(w198) -> ()
                    n77 = local write "SCM PROCESSES"(w191) -> ()
                    n78 = local write "VM PROCESSES"(w193) -> ()
                    n79 = local write "VP Cluster"(w182) -> ()
                    n80 = Unbundle By Name(w182) -> ("CA Output Numbers"=w179:i32[], "CA Input Numbers"=w178:i32[])
                    n81 = Unbundle By Name(w175) -> ("Input Numbers"=w174:i32[])
                    n82 = call "ParseAllBlocksMessages.vi"("Path"=w139) -> ("SCM2VM Msg Cluster Array"=w154:cluster{"Names":string[], "Codes":i32[]}, "VM INP from SCM Msg Cluster Array"=w158:cluster{"Names":string[], "Codes":i32[]}, "VM2SCM Msg Cluster Array"=w155:cluster{"Names":string[], "Codes":i32[]}, "COM2CA MSG Cluster Array"=w169:cluster{"Names":string[], "Codes":i32[]}, "SCM-SCM2VP Msg Cluster Array"=w150:cluster{"Names":string[], "Codes":i32[]}, "VP-SCM2VP Msg Cluster Array"=w149:cluster{"Names":string[], "Codes":i32[]}, "SCM2CA Msg Cluster Array"=w167:cluster{"Names":string[], "Codes":i32[]}, "CA2GUI Msg Cluster Array"=w164:cluster{"Names":string[], "Codes":i32[]}, "VM2GUI Msg Cluster Array"=w168:cluster{"Names":string[], "Codes":i32[]}, "VP 2 GUI Msg Cluster Array"=w138:cluster{"Names":string[], "Codes":i32[]}, "VM INP from CA Msg Cluster Array"=w163:cluster{"Names":string[], "Codes":i32[]}, "SCM - VM2SCM Msg Cluster Array"=w153:cluster{"Names":string[], "Codes":i32[]})  [unwired: 3 in]
                    n83 = local write "SCM2CA Msg Cluster Array"(w167) -> ()
                    n84 = local write "VM INP from SCM Msg Cluster Array"(w158) -> ()
                    n85 = Array Size(array=w181) -> (size(s)=w176:i32)
                    n86 = Array Size(array=w180) -> (size(s)=w177:i32)
                    n87 = local write "VP 2 GUI Msg Cluster Array"(w138) -> ()
                    n88 = Array Size(array=w179) -> (size(s)=w173:i32)
                    n89 = Array Size(array=w178) -> (size(s)=w172:i32)
                    n90 = local write "SCM2VM Msg Cluster Array"(w154) -> ()
                    n91 = local write "VM2SCM Msg Cluster Array"(w155) -> ()
                    n92 = local write "COM2CA MSG Cluster Array"(w169) -> ()
                    n93 = local write "CA2GUI Msg Cluster Array"(w164) -> ()
                    n94 = local write "SCM-SCM2VP Msg Cluster Array"(w150) -> ()
                    n95 = local write "VM2GUI Msg Cluster Array"(w168) -> ()
                    n96 = Array Size(array=w174) -> (size(s)=w170:i32)
                    n97 = Add(x=w173, y=w172) -> (x+y=w171:i32)
                    n98 = Equal?(x=w171, y=w170) -> (x = y?=w140:bool)
                    n99 = Unbundle By Name "БУС2ВОУ_"(w150) -> ("Names"=w151:string[])
                    n100 = Unbundle By Name "БВ2БУС_"(w155) -> ("Names"=w157:string[])
                    n101 = Unbundle By Name "БУС2ВОУ_"(w149) -> ("Names"=w152:string[])
                    n102 = Unbundle By Name "БВ2БУС_"(w153) -> ("Names"=w156:string[])
                    n103 = Equal?(x=w176, y=w172) -> (x = y?=w142:bool)
                    n104 = Equal?(x=w177, y=w173) -> (x = y?=w141:bool)
                    n105 = Unbundle By Name(w168) -> ("Names"=w186:string[], "Codes"=w184:i32[])
                    n106 = Unbundle By Name "БУС2БВ_"(w158) -> ("Names"=w160:string[])
                    n107 = Unbundle By Name "БУС2БВ_"(w154) -> ("Names"=w159:string[])
                    n108 = Unbundle By Name "КОМ2АУ_"(w167) -> ("Names"=w165:string[])
                    n109 = Unbundle By Name "КОМ2АУ_"(w169) -> ("Names"=w166:string[])
                    n110 = Equal?(x=w151, y=w152) -> (x = y?=w148:bool)
                    n111 = Equal?(x=w157, y=w156) -> (x = y?=w147:bool)
                    n112 = Array Size(array=w186) -> (size(s)=w185:i32)
                    n113 = while {
                      tunnel: w186 -> [w230] mode=indexing
                      tunnel: w185 -> [w227]
                      tunnel: w184 -> [w223] mode=indexing
                      i -> [w228]
                      stop <- w224 stop-if-true
                      n114 = To Lower Case(string=w230) -> (all lower case string=w229:string)
                      n115 = Equal?(x=w227, y=w228) -> (x = y?=w226:bool)
                      n116 = Search and Replace String(replace all?=FALSE ("replace all? (F)"), case sensitive?=TRUE ("ignore case? (F)"), input string=w229, search string="БВ2ГИО_ВерификацияЗавершена") -> (offset past replacement=w234:i32)  [unwired: 4 in, 3 out]
                      n117 = Less Than 0?(x=w234) -> (x < 0?=w235:bool)
                      n118 = case shown="False" w235 {
                        tunnel: [TRUE FALSE] -> w225
                        tunnel: w223 -> [w236 _]
                        frame False {
                          "End Number" <- w236
                        }
                        frame True {
                        }
                      }
                      n119 = Or(x=w225, y=w226) -> (x .or. y?=w224:bool)
                    }
                    n120 = Equal?(x=w160, y=w159) -> (x = y?=w146:bool)
                    n121 = Equal?(x=w166, y=w165) -> (x = y?=w144:bool)
                    n122 = Unbundle By Name "АУ2ГУИ_"(w164) -> ("Names"=w161:string[])
                    n123 = Unbundle By Name "АУ2ГУИ_"(w163) -> ("Names"=w162:string[])
                    n124 = Equal?(x=w161, y=w162) -> (x = y?=w145:bool)
                    n125 = Compound Arithmetic op=AND(w142, w141, w140, w148, w147, w146, w145, w144) -> (w143:bool)
                    n126 = case shown="True" w143 {
                      tunnel: w148 -> [w222 _]
                      tunnel: w147 -> [w221 _]
                      tunnel: w146 -> [w220 _]
                      tunnel: w145 -> [w219 _]
                      tunnel: w144 -> [w218 _]
                      tunnel: w142 -> [w205 _]
                      tunnel: w141 -> [w203 _]
                      tunnel: w140 -> [w202 _]
                      frame False {
                        n127 = Build Array(w205, w203, w202, w222, w221, w220, w219, w218) -> (w212:bool[])
                        n128 = Search 1D Array(1D array=w212, element=FALSE) -> (index of element=w209:i32)  [unwired: 1 in]
                        n129 = Build Array("Входные порты АУ и  выходные порты ВОУ", "Выходные порты АУ и  входные порты ВОУ", "Порты АУ, ВОУ и БВ", "БУС2ВОУ_", "БВ2БУС_", "БУС2БВ_", "АУ2ГУИ_", "КОМ2АУ_") -> (w210:string[])
                        n130 = Index Array(array=w210, index=w209) -> (element=w207:string)
                        n131 = Concatenate Strings("Ошибка загрузки алгоблоков! \nПроверьте соответствие следующих входных данных: " ("message"), w207) -> (w206:string)
                        n132 = One Button Dialog(message=w206) -> ()  [unwired: 1 in, 1 out]
                      }
                      frame True {
                      }
                    }
                  }
                }
              }
              frame #1 {
                n133 = case shown="True" w239 {
                  selector: w239 -> [_ w242]
                  frame False {
                  }
                  frame True {
                    n134 = flat-sequence {
                      tunnel: w242 -> [w246]
                      frame #0 {
                        n135 = local read "Проект"() -> (w244:path)
                        n136 = Path To String(path=w244) -> (string=w243:string)
                        n137 = dll-call lib="C:/Users/Татьяна Лях/Downloads/MyComplex-master/DLL-s/MakeFullImmitationStepDLL/Release/MakeFullImmitationStepDLL.dll" fn="?loadNewDlls@@YAHPAPAULabViewString@@@Z" label="Load NEW DLLs"("path"=w243) -> ("error"=→"error":i32)  [unwired: 4 in, 2 out]
                      }
                      frame #1 {
                        w249 = T8."Enabled" ("Disabled")
                        n138 = local write "Верификация запущена"(w246) -> ()
                        n139 = local write "Pause"(FALSE ("Pause")) -> ()
                        n140 = property on="Pause" class="Bool (strict)"("DisabledEnum"=w249) -> ()  [unwired: 2 in, 2 out]
                        n141 = property on="Stop Ver Button" class="Bool (strict)"("DisabledEnum"=w249) -> ()  [unwired: 2 in, 2 out]
                        n142 = property on="START Button" class="Bool (strict)"("DisabledEnum"=T8."Disabled and Grayed Out" ("Disabled")) -> ()  [unwired: 2 in, 2 out]
                      }
                    }
                  }
                }
                n143 = Send Notification(notification=enum16{"no command", "refresh"}."refresh", notifier=w241) -> ()  [unwired: 1 in, 2 out]
              }
            }
          }
        }
      }
      event "Pause": Mouse Down {
        n144 = event-data() -> ()  [unwired: 1 in, 7 out]
        n145 = local read "Верификация запущена"() -> (w251:bool)
        n146 = Not(x=w251) -> (.not. x?=w250:bool)
        n147 = local write "Верификация запущена"(w250) -> ()
      }
      event "Stop Ver Button": Mouse Down {
        n148 = event-data() -> ()  [unwired: 1 in, 7 out]
        n149 = flat-sequence {
          frame #0 {
            n150 = dll-call lib="C:/Users/Татьяна Лях/Downloads/MyComplex-master/DLL-s/MakeFullImmitationStepDLL/Release/MakeFullImmitationStepDLL.dll" fn="?freeAllDlls@@YAXXZ" label="FREE DLLs"() -> ()  [unwired: 4 in, 2 out]
          }
          frame #1 {
            w253 = T8."Disabled and Grayed Out" ("Disabled")
            n151 = local write "Pause"(FALSE ("Pause")) -> ()
            n152 = local write "Верификация запущена"(FALSE ("VerificationRunning")) -> ()
            n153 = property on="START Button" class="Bool (strict)"("DisabledEnum"=T8."Enabled" ("Disabled")) -> ()  [unwired: 2 in, 2 out]
            n154 = property on="Stop Ver Button" class="Bool (strict)"("DisabledEnum"=w253) -> ()  [unwired: 2 in, 2 out]
            n155 = property on="Pause" class="Bool (strict)"("DisabledEnum"=w253) -> ()  [unwired: 2 in, 2 out]
          }
        }
      }
      event Menu Selection (User) {
        n156 = event-data() -> ("MenuRef"=w257:refnum<k9>, "ItemTag"=w258:string)  [unwired: 1 in, 4 out]
        n157 = case shown="\"LoadIMG\"" w258 {
          tunnel: w257 -> [w260 w306 w307 w348 w352 w354]
          tunnel: [w260 w306 w307 w348 w352 w354] -> w256
          frame "New" {
            n158 = local read "Проект"() -> (w261:path)
            n159 = call "File Dialog2"("start path"=w261, "prompt"="Выберите папку, в которой хотите создать проект" ("default name"), "button label"="Создать проект в текущей папке" ("pattern label"), "default name"="Progect") -> ("selected path"=w264:path, "exists"=w263:bool, "cancelled"=w262:bool)  [unwired: 8 in, 1 out]
            "selected path" <- w264
            n160 = case shown="False" w262 {
              tunnel: w264 -> [w269 _]
              tunnel: w263 -> [w268 _]
              frame False {
                n161 = case shown="True" w268 {
                  tunnel: w269 -> [_ w270]
                  frame False {
                  }
                  frame True {
                    n162 = call "CreateNewProgect.vi"("selected path"=w270) -> ("Boolean"=w271:bool)
                    n163 = case shown="True" w271 {
                      selector: w271 -> [_ w304]
                      tunnel: w270 -> [_ w279]
                      frame False {
                      }
                      frame True {
                        w274 = T8."Disabled and Grayed Out" ("Disabled")
                        w284 = "Section 1" ("section")
                        w286 = path ""
                        n164 = Current VI's Menubar() -> (w276:refnum<k9>)
                        n165 = local write "Pause"(FALSE ("Pause")) -> ()
                        n166 = local write "Верификация запущена"(FALSE ("VerificationRunning")) -> ()
                        n167 = Strip Path(path=w279) -> (name=w280:string)  [unwired: 1 out]
                        n168 = local write "Project"(w280) -> ()
                        n169 = Set Menu Item Info(7:"LoadIMG" ("item tag"), 9:TRUE ("enabled"), 11:w276) -> ()  [unwired: 4 in, 2 out]
                        n170 = local write "Scalar"(w304) -> ()
                        n171 = Build Path(base path=w279, name or relative path="progect_cfg.ini") -> (appended path=w295:path)
                        n172 = call <vilib>:"Application Directory.vi"() -> ("Application Directory"=w303:path)
                        n173 = local write "Проект"(w279) -> ()
                        n174 = call <vilib>:"Open Config Data.vi"("create file if necessary (T)"=TRUE, "configuration file path"=w295) -> ("error out"=w293:errorcluster, "refnum"=w292:T9)  [unwired: 7 in, 1 out]
                        n175 = Build Path(base path=w303, name or relative path="cfg.ini") -> (appended path=w301:path)
                        n176 = local read "subpanel VI ref"() -> (w282:refnum<vi>)
                        n177 = call <vilib>:"Open Config Data.vi"("configuration file path"=w301) -> ("refnum"=w300:T9)  [unwired: 8 in, 2 out]
                        n178 = call-poly <vilib>:"Write Key.vi"("section"=w284, "error in (no error)"=w293, "value"=w286, "key"="pic", "refnum"=w292) -> ("error out"=w289:errorcluster, "refnum out"=w290:T9)  [unwired: 4 in, 1 out]
                        n179 = Equal?(x=w282, y=refnum<k0> refnum) -> (x = y?=w281:bool)
                        n180 = call-poly <vilib>:"Write Key.vi"("section"="Section 1", "value"=w279, "key"="Progect", "refnum"=w300) -> ("refnum out"=w297:T9)  [unwired: 5 in, 2 out]
                        n181 = case shown="False" w281 {
                          tunnel: w282 -> [w305 _]
                          frame False {
                            n182 = invoke on="Sub Panel" class="SubPnl" method="Remove VI"() -> ()  [unwired: 3 in, 3 out]
                            n183 = Close Reference(reference=w305) -> ()  [unwired: 1 in, 1 out]
                          }
                          frame True {
                          }
                        }
                        n184 = call-poly <vilib>:"Write Key.vi"("section"=w284, "error in (no error)"=w289, "value"=w286, "key"="xml", "refnum"=w290) -> ("error out"=w287:errorcluster, "refnum out"=w288:T9)  [unwired: 4 in, 1 out]
                        n185 = call <vilib>:"Close Config Data.vi"("refnum"=w297) -> ()  [unwired: 9 in, 2 out]
                        n186 = call <vilib>:"Close Config Data.vi"("error in (no error)"=w287, "refnum"=w288) -> ()  [unwired: 8 in, 2 out]
                        n187 = property on="START Button" class="Bool (strict)"("DisabledEnum"=T8."Enabled" ("Disabled")) -> ()  [unwired: 2 in, 2 out]
                        n188 = property on="Stop Ver Button" class="Bool (strict)"("DisabledEnum"=w274) -> ()  [unwired: 2 in, 2 out]
                        n189 = property on="Pause" class="Bool (strict)"("DisabledEnum"=w274) -> ()  [unwired: 2 in, 2 out]
                      }
                    }
                  }
                }
                "exists" <- w268
              }
              frame True {
              }
            }
          }
          frame Default {
          }
          frame "LoadIMG" {
            n190 = flat-sequence {
              frame #0 {
                n191 = local read "Проект"() -> (w308:path)
                n192 = call "File Dialog3"("start path"=w308, "prompt"="Выберите файл изображения", "pattern (all files)"="*.jpg; *.bmp; *.png") -> ("selected path"=w310:path, "cancelled"=w309:bool)  [unwired: 9 in, 2 out]
                n193 = case shown="False" w309 {
                  tunnel: w310 -> [w315 _]
                  tunnel: w308 -> [w313 _]
                  frame False {
                    n194 = call "File Dialog4"("start path"=w313, "prompt"="Выберите файл XML", "pattern (all files)"="*.xml") -> ("selected path"=w318:path, "cancelled"=w314:bool)  [unwired: 9 in, 2 out]
                    n195 = case shown="False" w314 {
                      tunnel: w318 -> [w320 _]
                      tunnel: w315 -> [w319 _]
                      frame False {
                        n196 = local read "Проект"() -> (w321:path)
                        n197 = flat-sequence {
                          tunnel: w321 -> [w325]
                          tunnel: w320 -> [w324]
                          tunnel: w319 -> [w323]
                          tunnel: w321 -> [w343]
                          frame #0 {
                            w334 = "Section 1" ("section")
                            n198 = Build Path(base path=w325, name or relative path="progect_cfg.ini") -> (appended path=w326:path)
                            n199 = call <vilib>:"Open Config Data.vi"("create file if necessary (T)"=TRUE, "configuration file path"=w326) -> ("error out"=w328:errorcluster, "refnum"=w329:T9)  [unwired: 7 in, 1 out]
                            n200 = call-poly <vilib>:"Write Key.vi"("section"=w334, "error in (no error)"=w328, "value"=w323, "key"="pic", "refnum"=w329) -> ("error out"=w333:errorcluster, "refnum out"=w336:T9)  [unwired: 4 in, 1 out]
                            n201 = call-poly <vilib>:"Write Key.vi"("section"=w334, "error in (no error)"=w333, "value"=w324, "key"="xml", "refnum"=w336) -> ("error out"=w331:errorcluster, "refnum out"=w335:T9)  [unwired: 4 in, 1 out]
                            n202 = call <vilib>:"Close Config Data.vi"("error in (no error)"=w331, "refnum"=w335) -> ()  [unwired: 8 in, 2 out]
                          }
                          frame #1 {
                            n203 = local read "subpanel VI ref"() -> (w337:refnum<vi>)
                            n204 = Equal?(x=w337, y=refnum<k0> refnum) -> (x = y?=w338:bool)
                            n205 = case shown="False" w338 {
                              tunnel: w337 -> [w340 _]
                              frame False {
                                n206 = invoke on="Sub Panel" class="SubPnl" method="Remove VI"() -> (error out=w341:errorcluster)  [unwired: 3 in, 2 out]
                                n207 = Close Reference(reference=w340, error in (no error)=w341) -> ()  [unwired: 1 out]
                              }
                              frame True {
                              }
                            }
                          }
                          frame #2 {
                            n208 = control-ref of="algInputPorts"() -> ()  [unwired: 1 out]
                            n209 = control-ref of="algOutputPorts"() -> ()  [unwired: 1 out]
                            n210 = call "Load PIC and XML.vi"("selected path"=w343) -> ("toChanger"=w342:T1, "vi refnum"=w346:refnum<vi>)  [unwired: 2 in]
                            n211 = local write "toChanger"(w342) -> ()
                            n212 = Equal?(x=refnum<k0> refnum, y=w346) -> (x = y?=w345:bool)
                            n213 = case shown="False" w345 {
                              tunnel: w346 -> [w347 _]
                              frame False {
                                n214 = invoke on="Sub Panel" class="SubPnl" method="Insert VI"("VI Ref"=w347) -> ()  [unwired: 3 in, 4 out]
                              }
                              frame True {
                              }
                            }
                          }
                        }
                      }
                      frame True {
                      }
                    }
                  }
                  frame True {
                  }
                }
              }
            }
          }
          frame "ProjDescr" {
            n215 = local read "Проект"() -> (w349:path)
            n216 = call <vilib>:"System Exec.vi"("wait until completion? (T)"=FALSE, "working directory"=w349, "command line"="C:\\Program Files (x86)\\Notepad++\\notepad++.exe  \"Описание проекта.txt\"" ("name or relative path")) -> ()  [unwired: 5 in, 4 out]
          }
          frame "About" {
            n217 = One Button Dialog(message="Описание программы.\n\nКомплекс автоматической верификации промышленных алгоритмов управления.\n\nНачало работы:\n\n1)\tПроект -> Создать проект -> Создать проект в текущей директории. \nПосле этого в выбранной директории создадутся папки:\n- CA\n- VP \n- SCM\n- VM\nВ каждой папке появятся файлы-заготовки RCS с шаблоном кода на языке Reflex\n2)\tКнопка Редактирование открывает редактор с .rcs файлами.\n3)\tПосле редактирования кода на языке Reflex запускаем скрипт BUILD\n4)\tВывод скрипта делится на две части: Вывод транслятора из языка Reflex в язык C и вывод компилятора. \nВывод транслятора: Если пишется, что PASS ONE COMPLETE. PASS TWO COMPLETE. - Значит, ошибок в коде на языке Reflex нет.\nВывод компилятора - стандартный вывоз компилятора  GCC. Если ошибок нет и появляется строчка Скопировано файлов - 1, то ошибок при создании DLL нет. \n5)\tЕсли нет ошибок и DLL сгенерировано, можно приступать к верификации.\nВ окне \"Окно верификации\" Нажмите кнопку запуска верификации. Верификация началась.\nСостояние алгоблоков можно проверить, открыв панели состояний алгоблоков БУС, БУВ, ВОУ И АУ.\n\nПо завершению верификации появится сообщение \"Верификация завершена!\"\n\nТребуемые префиксы сообщений алгоблоков:\nАУ:\n- КОМ2АУ_ - входные сообщения алгоритма;\n- АУ2ГИО_ - выходные сообщения алгоритма;\nВОУ:\n- БУС2ВОУ_ - входные сообщения от блока управления сценариями имитатору объекта \n- ВОУ2ГИО_ - выходные сообщения от объекта управления\nБУС:\n- БУС2ВОУ_ - выходные команды объекту управления\n- КОМ2АУ_ - выходные сообщения алгоритму\n- БУС2БВ_ - выходные сообщения верификатору\n- БВ2БУС_ - входные сообщения от верификатора\nБВ:\n- АУ2ГИО__ - выходные сообщения алгоритма;\n- БУС2БВ_ - входные сообщения от БУС\n- БВ2БУС_ - выходные сообщения от для БВ\n- БВ2ГИО_ = выходные команды для ГИО\n  ") -> ()  [unwired: 1 in, 1 out]
          }
          frame "Open" {
            n218 = call <vilib>:"Application Directory.vi"() -> ("Application Directory"=w358:path)
            n219 = call "File Dialog"("start path"=w358, "prompt"="Выбрать файл проекта" ("default name"), "button label"="Выбрать проект" ("pattern label")) -> ("selected path"=w355:path, "cancelled"=w356:bool)  [unwired: 9 in, 2 out]
            n220 = case shown="False" w356 {
              tunnel: w355 -> [w360 _]
              frame False {
                n221 = List Folder(path=w360) -> (folder names=w370:string[])  [unwired: 3 in, 3 out]
                n222 = Search 1D Array(1D array=w370, element="VP") -> (index of element=w367:i32)  [unwired: 1 in]
                n223 = Search 1D Array(1D array=w370, element="CA") -> (index of element=w368:i32)  [unwired: 1 in]
                n224 = Search 1D Array(1D array=w370, element="VM") -> (index of element=w365:i32)  [unwired: 1 in]
                n225 = Search 1D Array(1D array=w370, element="SCM") -> (index of element=w366:i32)  [unwired: 1 in]
                n226 = Build Array(w368, w367, w366, w365) -> (w364:i32[])
                n227 = call "Convert to Dynamic Data"("Array"=w364) -> ("Dynamic Data Type"=w363:dynamicdata)  [unwired: 3 in]
                n228 = call "Greater or Equal"("Constant Value to Compare Against"=0, "Operand 1"=w363) -> ("Result"=w362:dynamicdata)  [unwired: 8 in, 1 out]
                n229 = call "Convert from Dynamic Data"("Dynamic Data Type"=w362) -> ("Scalar"=w361:bool)  [unwired: 3 in]
                "Scalar" <- w361
                n230 = case shown="True" w361 {
                  tunnel: w360 -> [_ w380]
                  frame False {
                    n231 = One Button Dialog(message="Wrong progect path!") -> ()  [unwired: 1 in, 1 out]
                  }
                  frame True {
                    w378 = T8."Disabled and Grayed Out" ("Disabled")
                    n232 = flat-sequence {
                      tunnel: w380 -> [w397]
                      tunnel: [w397] -> w381
                      tunnel: w381 -> [w400]
                      frame #0 {
                        n233 = local read "subpanel VI ref"() -> (w394:refnum<vi>)
                        n234 = Equal?(x=w394, y=refnum<k0> refnum) -> (x = y?=w395:bool)
                        n235 = case shown="False" w395 {
                          tunnel: w394 -> [w398 _]
                          frame False {
                            n236 = invoke on="Sub Panel" class="SubPnl" method="Remove VI"() -> ()  [unwired: 3 in, 3 out]
                            n237 = Close Reference(reference=w398) -> ()  [unwired: 1 in, 1 out]
                          }
                          frame True {
                          }
                        }
                      }
                      frame #1 {
                        n238 = call "Load PIC and XML.vi"("selected path"=w400) -> ("toChanger"=w399:T1, "vi refnum"=w401:refnum<vi>)  [unwired: 2 in]
                        n239 = local write "toChanger"(w399) -> ()
                        n240 = Equal?(x=refnum<k0> refnum, y=w401) -> (x = y?=w402:bool)
                        n241 = case shown="False" w402 {
                          tunnel: w401 -> [w404 _]
                          frame False {
                            n242 = invoke on="Sub Panel" class="SubPnl" method="Insert VI"("VI Ref"=w404) -> ()  [unwired: 3 in, 4 out]
                          }
                          frame True {
                          }
                        }
                      }
                    }
                    n243 = property on="START Button" class="Bool (strict)"("DisabledEnum"=T8."Enabled" ("Disabled")) -> ()  [unwired: 2 in, 2 out]
                    n244 = local write "Pause"(FALSE ("Pause")) -> ()
                    n245 = local write "Верификация запущена"(FALSE ("VerificationRunning")) -> ()
                    n246 = property on="Stop Ver Button" class="Bool (strict)"("DisabledEnum"=w378) -> ()  [unwired: 2 in, 2 out]
                    n247 = property on="Pause" class="Bool (strict)"("DisabledEnum"=w378) -> ()  [unwired: 2 in, 2 out]
                    n248 = local write "Проект"(w380) -> ()
                    n249 = Strip Path(path=w380) -> (name=w393:string)  [unwired: 1 out]
                    n250 = local read "Проект"() -> (w385:path)
                    n251 = call <vilib>:"Application Directory.vi"() -> ("Application Directory"=w392:path)
                    n252 = Current VI's Menubar() -> (w384:refnum<k9>)
                    n253 = local write "Project"(w393) -> ()
                    n254 = Build Path(base path=w392, name or relative path="cfg.ini") -> (appended path=w390:path)
                    n255 = call <vilib>:"Open Config Data.vi"("configuration file path"=w390) -> ("refnum"=w389:T9)  [unwired: 8 in, 2 out]
                    n256 = call-poly <vilib>:"Write Key.vi"("section"="Section 1", "value"=w385, "key"="Progect", "refnum"=w389) -> ("refnum out"=w387:T9)  [unwired: 5 in, 2 out]
                    n257 = Set Menu Item Info(7:"LoadIMG" ("item tag"), 9:TRUE ("enabled"), 11:w384) -> ()  [unwired: 4 in, 2 out]
                    n258 = call <vilib>:"Close Config Data.vi"("refnum"=w387) -> ()  [unwired: 9 in, 2 out]
                  }
                }
              }
              frame True {
              }
            }
          }
        }
        n259 = Enable Menu Tracking(3:TRUE ("enable (T)"), 4:w256) -> ()  [unwired: 1 in, 2 out]
      }
      event "Открыть панель АУ": Mouse Up {
        n260 = event-data() -> ()  [unwired: 1 in, 7 out]
        n261 = local read "CA vi reference"() -> (w447:refnum<vi>)
        n262 = invoke class="VI" method="FP.Open"(reference=w447) -> (reference out=w446:refnum<vi>, error out=w444:errorcluster)  [unwired: 4 in, 3 out]
        n263 = control-ref of="CA DESCR"() -> (w443:refnum<vi>)
        n264 = invoke class="VI" method="Ctrl Val.Set"(reference=w446, error in=w444, "Control Name"="PORTS", "Value"=w443) -> (reference out=w442:refnum<vi>, error out=w441:errorcluster)  [unwired: 1 in, 3 out]
        n265 = control-ref of="algInputPorts"() -> (w439:refnum<vi>)
        n266 = invoke class="VI" method="Ctrl Val.Set"(reference=w442, error in=w441, "Control Name"="INP", "Value"=w439) -> (reference out=w437:refnum<vi>, error out=w436:errorcluster)  [unwired: 1 in, 3 out]
        n267 = control-ref of="algOutputPorts"() -> (w435:refnum<vi>)
        n268 = invoke class="VI" method="Ctrl Val.Set"(reference=w437, error in=w436, "Control Name"="OUTP", "Value"=w435) -> (reference out=w432:refnum<vi>, error out=w431:errorcluster)  [unwired: 1 in, 3 out]
        n269 = control-ref of="CA PROCESSES"() -> (w425:refnum<vi>)
        n270 = invoke class="VI" method="Ctrl Val.Set"(reference=w432, error in=w431, "Control Name"="Processes", "Value"=w425) -> (reference out=w430:refnum<vi>, error out=w429:errorcluster)  [unwired: 1 in, 3 out]
        n271 = control-ref of="CA STATES"() -> (w424:refnum<vi>)
        n272 = invoke class="VI" method="Ctrl Val.Set"(reference=w430, error in=w429, "Control Name"="States", "Value"=w424) -> (reference out=w427:refnum<vi>, error out=w426:errorcluster)  [unwired: 1 in, 3 out]
        n273 = control-ref of="algStates"() -> (w423:refnum<vi>)
        n274 = invoke class="VI" method="Ctrl Val.Set"(reference=w427, error in=w426, "Control Name"="AlgStates", "Value"=w423) -> (reference out=w422:refnum<vi>, error out=w421:errorcluster)  [unwired: 1 in, 3 out]
        n275 = control-ref of="CA2GUI Msg Cluster Array"() -> (w405:refnum<vi>)
        n276 = invoke class="VI" method="Ctrl Val.Set"(reference=w422, error in=w421, "Control Name"="CA2GUI", "Value"=w405) -> (reference out=w419:refnum<vi>, error out=w418:errorcluster)  [unwired: 1 in, 3 out]
        n277 = control-ref of="algOutputMsgs"() -> (w417:refnum<vi>)
        n278 = invoke class="VI" method="Ctrl Val.Set"(reference=w419, error in=w418, "Control Name"="algOutputMsgs", "Value"=w417) -> (reference out=w414:refnum<vi>, error out=w413:errorcluster)  [unwired: 1 in, 3 out]
        n279 = control-ref of="CA input vars"() -> (w412:refnum<vi>)
        n280 = invoke class="VI" method="Ctrl Val.Set"(reference=w414, error in=w413, "Control Name"="INPUT VARS", "Value"=w412) -> (reference out=w411:refnum<vi>, error out=w410:errorcluster)  [unwired: 1 in, 3 out]
        n281 = control-ref of="CA output vars"() -> (w406:refnum<vi>)
        n282 = invoke class="VI" method="Ctrl Val.Set"(reference=w411, error in=w410, "Control Name"="OUTPUT VARS", "Value"=w406) -> (reference out=w409:refnum<vi>, error out=w408:errorcluster)  [unwired: 1 in, 3 out]
        n283 = invoke class="VI" method="Run VI"(reference=w409, error in=w408, "Wait until done"=FALSE ("Wait Until Done")) -> (error out=→"error out":errorcluster)  [unwired: 2 in, 4 out]
      }
      event "Открыть панель ВОУ": Mouse Up {
        n284 = event-data() -> ()  [unwired: 1 in, 7 out]
        n285 = local read "VP vi reference"() -> (w491:refnum<vi>)
        n286 = invoke class="VI" method="FP.Open"(reference=w491) -> (reference out=w463:refnum<vi>)  [unwired: 4 in, 4 out]
        n287 = control-ref of="VP Cluster"() -> (w454:refnum<vi>)
        n288 = invoke class="VI" method="Ctrl Val.Set"(reference=w463, "Control Name"="PORTS", "Value"=w454) -> (reference out=w489:refnum<vi>, error out=w488:errorcluster)  [unwired: 2 in, 3 out]
        n289 = control-ref of="algOutputPorts"() -> (w461:refnum<vi>)
        n290 = invoke class="VI" method="Ctrl Val.Set"(reference=w489, error in=w488, "Control Name"="INP", "Value"=w461) -> (reference out=w485:refnum<vi>, error out=w484:errorcluster)  [unwired: 1 in, 3 out]
        n291 = control-ref of="algInputPorts"() -> (w460:refnum<vi>)
        n292 = invoke class="VI" method="Ctrl Val.Set"(reference=w485, error in=w484, "Control Name"="OUTP", "Value"=w460) -> (reference out=w481:refnum<vi>, error out=w480:errorcluster)  [unwired: 1 in, 3 out]
        n293 = control-ref of="VP PROCESSES"() -> (w459:refnum<vi>)
        n294 = invoke class="VI" method="Ctrl Val.Set"(reference=w481, error in=w480, "Control Name"="Processes", "Value"=w459) -> (reference out=w479:refnum<vi>, error out=w478:errorcluster)  [unwired: 1 in, 3 out]
        n295 = control-ref of="VP STATES"() -> (w458:refnum<vi>)
        n296 = invoke class="VI" method="Ctrl Val.Set"(reference=w479, error in=w478, "Control Name"="States", "Value"=w458) -> (reference out=w476:refnum<vi>, error out=w475:errorcluster)  [unwired: 1 in, 3 out]
        n297 = control-ref of="vplantStates"() -> (w457:refnum<vi>)
        n298 = invoke class="VI" method="Ctrl Val.Set"(reference=w476, error in=w475, "Control Name"="VPStates", "Value"=w457) -> (reference out=w474:refnum<vi>, error out=w473:errorcluster)  [unwired: 1 in, 3 out]
        n299 = control-ref of="VP 2 GUI Msg Cluster Array"() -> (w453:refnum<vi>)
        n300 = invoke class="VI" method="Ctrl Val.Set"(reference=w474, error in=w473, "Control Name"="VP2GUI", "Value"=w453) -> (reference out=w471:refnum<vi>, error out=w470:errorcluster)  [unwired: 1 in, 3 out]
        n301 = control-ref of="virtualPlant2GUIOutputMsgs"() -> (w451:refnum<vi>)
        n302 = invoke class="VI" method="Ctrl Val.Set"(reference=w471, error in=w470, "Control Name"="VPOutputMsgs", "Value"=w451) -> (reference out=w468:refnum<vi>, error out=w467:errorcluster)  [unwired: 1 in, 3 out]
        n303 = control-ref of="VP input vars"() -> (w456:refnum<vi>)
        n304 = invoke class="VI" method="Ctrl Val.Set"(reference=w468, error in=w467, "Control Name"="INPUT VARS", "Value"=w456) -> (reference out=w466:refnum<vi>, error out=w465:errorcluster)  [unwired: 1 in, 3 out]
        n305 = control-ref of="VP output vars"() -> (w455:refnum<vi>)
        n306 = invoke class="VI" method="Ctrl Val.Set"(reference=w466, error in=w465, "Control Name"="OUTPUT VARS", "Value"=w455) -> (reference out=w462:refnum<vi>)  [unwired: 1 in, 4 out]
        n307 = invoke class="VI" method="Run VI"(reference=w462, "Wait until done"=FALSE ("Wait Until Done")) -> (error out=w450:errorcluster)  [unwired: 3 in, 4 out]
        n308 = local write "error out"(w450) -> ()
      }
      event "Открыть панель БУС": Mouse Up {
        n309 = event-data() -> ()  [unwired: 1 in, 7 out]
        n310 = local read "SCB vi reference"() -> (w532:refnum<vi>)
        n311 = invoke class="VI" method="FP.Open"(reference=w532) -> (reference out=w522:refnum<vi>, error out=w523:errorcluster)  [unwired: 4 in, 3 out]
        n312 = control-ref of="SCM PROCESSES"() -> (w501:refnum<vi>)
        n313 = invoke class="VI" method="Ctrl Val.Set"(reference=w522, error in=w523, "Control Name"="Processes", "Value"=w501) -> (reference out=w528:refnum<vi>, error out=w527:errorcluster)  [unwired: 1 in, 3 out]
        n314 = control-ref of="SCM STATES"() -> (w500:refnum<vi>)
        n315 = invoke class="VI" method="Ctrl Val.Set"(reference=w528, error in=w527, "Control Name"="States", "Value"=w500) -> (reference out=w525:refnum<vi>, error out=w524:errorcluster)  [unwired: 1 in, 3 out]
        n316 = control-ref of="scenarioStates"() -> (w499:refnum<vi>)
        n317 = invoke class="VI" method="Ctrl Val.Set"(reference=w525, error in=w524, "Control Name"="SCBStates", "Value"=w499) -> (reference out=w517:refnum<vi>, error out=w516:errorcluster)  [unwired: 1 in, 3 out]
        n318 = control-ref of="SCM2VM Msg Cluster Array"() -> (w498:refnum<vi>)
        n319 = invoke class="VI" method="Ctrl Val.Set"(reference=w517, error in=w516, "Control Name"="SCM2VM", "Value"=w498) -> (reference out=w519:refnum<vi>, error out=w518:errorcluster)  [unwired: 1 in, 3 out]
        n320 = control-ref of="scenarios2VerifierOutputMsgs"() -> (w494:refnum<vi>)
        n321 = invoke class="VI" method="Ctrl Val.Set"(reference=w519, error in=w518, "Control Name"="VMInputMsgs", "Value"=w494) -> (reference out=w511:refnum<vi>, error out=w510:errorcluster)  [unwired: 1 in, 3 out]
        n322 = control-ref of="SCM-SCM2VP Msg Cluster Array"() -> (w497:refnum<vi>)
        n323 = invoke class="VI" method="Ctrl Val.Set"(reference=w511, error in=w510, "Control Name"="SCM2VP", "Value"=w497) -> (reference out=w513:refnum<vi>, error out=w512:errorcluster)  [unwired: 1 in, 3 out]
        n324 = control-ref of="scenarios2VirtPlantOutputMsgs"() -> (w493:refnum<vi>)
        n325 = invoke class="VI" method="Ctrl Val.Set"(reference=w513, error in=w512, "Control Name"="VPInputMsgs", "Value"=w493) -> (reference out=w505:refnum<vi>, error out=w504:errorcluster)  [unwired: 1 in, 3 out]
        n326 = control-ref of="SCM2CA Msg Cluster Array"() -> (w496:refnum<vi>)
        n327 = invoke class="VI" method="Ctrl Val.Set"(reference=w505, error in=w504, "Control Name"="SCM2CA", "Value"=w496) -> (reference out=w507:refnum<vi>, error out=w506:errorcluster)  [unwired: 1 in, 3 out]
        n328 = control-ref of="scenarios2AlgOutputMsgs"() -> (w495:refnum<vi>)
        n329 = invoke class="VI" method="Ctrl Val.Set"(reference=w507, error in=w506, "Control Name"="СAInputMsgs", "Value"=w495) -> (reference out=w503:refnum<vi>, error out=w502:errorcluster)  [unwired: 1 in, 3 out]
        n330 = invoke class="VI" method="Run VI"(reference=w503, error in=w502, "Wait until done"=FALSE ("Wait Until Done")) -> (error out=w531:errorcluster)  [unwired: 2 in, 4 out]
        n331 = local write "error out"(w531) -> ()
      }
      event "Открыть панель БВ": Mouse Up {
        n332 = event-data() -> ()  [unwired: 1 in, 7 out]
        n333 = local read "VM vi reference"() -> (w588:refnum<vi>)
        n334 = invoke class="VI" method="FP.Open"(reference=w588) -> (reference out=w580:refnum<vi>)  [unwired: 4 in, 4 out]
        n335 = control-ref of="VM PROCESSES"() -> (w578:refnum<vi>)
        n336 = invoke class="VI" method="Ctrl Val.Set"(reference=w580, "Control Name"="Processes", "Value"=w578) -> (reference out=w585:refnum<vi>, error out=w584:errorcluster)  [unwired: 2 in, 3 out]
        n337 = control-ref of="VM STATES"() -> (w577:refnum<vi>)
        n338 = invoke class="VI" method="Ctrl Val.Set"(reference=w585, error in=w584, "Control Name"="States", "Value"=w577) -> (reference out=w582:refnum<vi>, error out=w581:errorcluster)  [unwired: 1 in, 3 out]
        n339 = control-ref of="verStates"() -> (w579:refnum<vi>)
        n340 = invoke class="VI" method="Ctrl Val.Set"(reference=w582, error in=w581, "Control Name"="VMStates", "Value"=w579) -> (reference out=w572:refnum<vi>, error out=w571:errorcluster)  [unwired: 1 in, 3 out]
        n341 = control-ref of="VM DESCR"() -> (w567:refnum<vi>)
        n342 = invoke class="VI" method="Ctrl Val.Set"(reference=w572, error in=w571, "Control Name"="PORTS", "Value"=w567) -> (reference out=w575:refnum<vi>, error out=w574:errorcluster)  [unwired: 1 in, 3 out]
        n343 = control-ref of="algInputPorts"() -> (w566:refnum<vi>)
        n344 = invoke class="VI" method="Ctrl Val.Set"(reference=w575, error in=w574, "Control Name"="INP", "Value"=w566) -> (reference out=w569:refnum<vi>, error out=w568:errorcluster)  [unwired: 1 in, 3 out]
        n345 = control-ref of="algOutputPorts"() -> (w565:refnum<vi>)
        n346 = invoke class="VI" method="Ctrl Val.Set"(reference=w569, error in=w568, "Control Name"="OUTP", "Value"=w565) -> (reference out=w563:refnum<vi>, error out=w562:errorcluster)  [unwired: 1 in, 3 out]
        n347 = control-ref of="VM input vars"() -> (w561:refnum<vi>)
        n348 = invoke class="VI" method="Ctrl Val.Set"(reference=w563, error in=w562, "Control Name"="INPUT VARS", "Value"=w561) -> (reference out=w550:refnum<vi>, error out=w549:errorcluster)  [unwired: 1 in, 3 out]
        n349 = control-ref of="CA2GUI Msg Cluster Array"() -> (w547:refnum<vi>)
        n350 = invoke class="VI" method="Ctrl Val.Set"(reference=w550, error in=w549, "Control Name"="CA2GUI", "Value"=w547) -> (reference out=w552:refnum<vi>, error out=w553:errorcluster)  [unwired: 1 in, 3 out]
        n351 = control-ref of="algOutputMsgs"() -> (w548:refnum<vi>)
        n352 = invoke class="VI" method="Ctrl Val.Set"(reference=w552, error in=w553, "Control Name"="algOutputMsgs", "Value"=w548) -> (reference out=w556:refnum<vi>, error out=w557:errorcluster)  [unwired: 1 in, 3 out]
        n353 = control-ref of="VM2GUI Msg Cluster Array"() -> (w546:refnum<vi>)
        n354 = invoke class="VI" method="Ctrl Val.Set"(reference=w556, error in=w557, "Control Name"="VM2GUI", "Value"=w546) -> (reference out=w559:refnum<vi>, error out=w560:errorcluster)  [unwired: 1 in, 3 out]
        n355 = control-ref of="verifier2GUIOutputMsgs"() -> (w545:refnum<vi>)
        n356 = invoke class="VI" method="Ctrl Val.Set"(reference=w559, error in=w560, "Control Name"="verifier2GUIOutputMsgs", "Value"=w545) -> (reference out=w541:refnum<vi>, error out=w540:errorcluster)  [unwired: 1 in, 3 out]
        n357 = control-ref of="VM2SCM Msg Cluster Array"() -> (w539:refnum<vi>)
        n358 = invoke class="VI" method="Ctrl Val.Set"(reference=w541, error in=w540, "Control Name"="VM2SCM", "Value"=w539) -> (reference out=w543:refnum<vi>, error out=w542:errorcluster)  [unwired: 1 in, 3 out]
        n359 = control-ref of="verifier2scenariousControlOutMsgs"() -> (w537:refnum<vi>)
        n360 = invoke class="VI" method="Ctrl Val.Set"(reference=w543, error in=w542, "Control Name"="verifier2scenariousControlOutMsgs", "Value"=w537) -> (reference out=w536:refnum<vi>, error out=w535:errorcluster)  [unwired: 1 in, 3 out]
        n361 = invoke class="VI" method="Run VI"(reference=w536, error in=w535, "Wait until done"=FALSE ("Wait Until Done")) -> (error out=w534:errorcluster)  [unwired: 2 in, 4 out]
        n362 = local write "error out"(w534) -> ()
      }
      event "stop": Mouse Down {
        n363 = event-data() -> ()  [unwired: 1 in, 7 out]
        n364 = Open Application Reference() -> (3:w590:refnum<vi>)  [unwired: 4 in, 1 out]
        n365 = property class="App"(reference=w590) -> (error out=w592:errorcluster, "App.AllVIs"=w591:string[])  [unwired: 1 in, 1 out]
        n366 = dll-call lib="C:/Users/Татьяна Лях/Downloads/MyComplex-master/DLL-s/MakeFullImmitationStepDLL/Release/MakeFullImmitationStepDLL.dll" fn="?freeAllDlls@@YAXXZ" label="FREE DLLs"() -> ()  [unwired: 4 in, 2 out]
        n367 = for {
          tunnel: w591 -> [w596] mode=indexing
          tunnel: w592 -> [w601]
          n368 = Open VI Reference(vi path=w596, error in (no error)=w601) -> (vi reference=w600:refnum<vi>, error out=w599:errorcluster)  [unwired: 4 in]
          n369 = property class="VI"(reference=w600, error in=w599) -> (reference out=w597:refnum<vi>, error out=w595:errorcluster, "Front Panel.Open"=w598:bool)
          n370 = Unbundle By Name(w595) -> ("status"=w594:bool)
          n371 = case shown="True" w594 {
            tunnel: w598 -> [w604 _]
            tunnel: w597 -> [w603 _]
            frame False {
              n372 = case shown="True" w604 {
                tunnel: w603 -> [w605 w607]
                tunnel: [w605 w606] -> w602
                frame False {
                }
                frame True {
                  n373 = invoke class="VI" method="FP.Close"(reference=w607) -> (reference out=w606:refnum<vi>)  [unwired: 2 in, 2 out]
                }
              }
              n374 = Close Reference(reference=w602) -> ()  [unwired: 1 in, 1 out]
            }
            frame True {
            }
          }
        }
        n375 = flat-sequence {
          frame #0 {
            n376 = invoke on="Sub Panel" class="SubPnl" method="Remove VI"() -> ()  [unwired: 3 in, 3 out]
          }
          frame #1 {
            n377 = local read "subpanel VI ref"() -> (w593:refnum<vi>)
            n378 = Close Reference(reference=w593) -> ()  [unwired: 1 in, 1 out]
          }
        }
      }
      event Application Instance Close {
        n379 = event-data() -> ()  [unwired: 1 in, 3 out]
        n380 = dll-call lib="C:/Users/Татьяна Лях/Downloads/MyComplex-master/DLL-s/MakeFullImmitationStepDLL/Release/MakeFullImmitationStepDLL.dll" fn="?freeAllDlls@@YAXXZ" label="FREE DLLs"() -> ()  [unwired: 4 in, 2 out]
      }
    }
    n381 = local read "Верификация запущена"() -> (→"Verification":bool)
    n382 = local read "Верификация запущена"() -> (w46:bool)
    n383 = case shown="True" w46 {
      tunnel: "Режим работы:" -> [_ w78]
      frame False {
      }
      frame True {
        n384 = Boolean To (0,1)(Boolean=w78) -> (0, 1=w77:i16)
        n385 = dll-call lib="C:/Users/Татьяна Лях/Downloads/MyComplex-master/DLL-s/MakeFullImmitationStepDLL/Release/MakeFullImmitationStepDLL.dll" fn="?setMode@@YAXE@Z" label="setMode"("mode"=w77) -> (error out=w76:errorcluster)  [unwired: 5 in, 1 out]
        n386 = dll-call lib="C:/Users/Татьяна Лях/Downloads/MyComplex-master/DLL-s/MakeFullImmitationStepDLL/Release/MakeFullImmitationStepDLL.dll" fn="?LLD@@YAHPAPAUPort@@0PAPAUArrayOfMessages@@111111PAPAUArrayOfStates@@222@Z" label="Init"(error in=w76, "algInputPorts"="algInputPorts", "algOutputPorts"="algOutputPorts", "scenarios2AlgOutputMsgs"="scenarios2AlgOutputMsgs", "scenarios2VirtPlantOutputMsgs"="scenarios2VirtPlantOutputMsgs", "scenarios2VerifierOutputMsgs"="scenarios2VerifierOutputMsgs", "verifier2scenariousControlOutMsgs,"="verifier2scenariousControlOutMsgs", "algOutputMsgs"="algOutputMsgs", "verifier2GUIOutputMsgs"="verifier2GUIOutputMsgs", "virtualPlant2GUIOutputMsgs"="virtualPlant2GUIOutputMsgs", "algStates"="algStates", "vplantStates"="vplantStates", "verStates"="verStates", "scenarioStates"="scenarioStates") -> ("algInputPorts"=w50:i8[], "algOutputPorts"=w49:i8[], "scenarios2AlgOutputMsgs"=w58:cluster{"MSG":i16, "param":i32, "Type":i16}[], "scenarios2VirtPlantOutputMsgs"=w56:cluster{"MSG":i16, "param":i32, "Type":i16}[], "scenarios2VerifierOutputMsgs"=w57:cluster{"MSG":i16, "param":i32, "Type":i16}[], "verifier2scenariousControlOutMsgs,"=w54:cluster{"MSG":i16, "param":i32, "Type":i16}[], "algOutputMsgs"=w61:T7, "verifier2GUIOutputMsgs"=w52:cluster{"MSG":i16, "param":i32, "Type":i16}[], "virtualPlant2GUIOutputMsgs"=w60:cluster{"MSG":i16, "param":i32, "Type":i16}[], "algStates"=w62:cluster{"TimeInState":u16, "cur_state":i8}[], "vplantStates"=w59:cluster{"TimeInState":u16, "cur_state":i8}[], "verStates"=w53:cluster{"TimeInState":u16, "cur_state":i8}[], "scenarioStates"=w55:cluster{"TimeInState":u16, "cur_state":i8}[])  [unwired: 3 in, 2 out]
        n387 = local write "scenarioStates"(w55) -> ()
        n388 = local write "verStates"(w53) -> ()
        n389 = local write "virtualPlant2GUIOutputMsgs"(w60) -> ()
        n390 = local write "verifier2GUIOutputMsgs"(w52) -> ()
        n391 = local write "algInputPorts"(w50) -> ()
        n392 = local write "algOutputPorts"(w49) -> ()
        n393 = local write "verifier2scenariousControlOutMsgs"(w54) -> ()
        n394 = local write "vplantStates"(w59) -> ()
        n395 = local write "algStates"(w62) -> ()
        n396 = local write "algOutputMsgs"(w61) -> ()
        n397 = local write "scenarios2VirtPlantOutputMsgs"(w56) -> ()
        n398 = local write "scenarios2VerifierOutputMsgs"(w57) -> ()
        n399 = local write "scenarios2AlgOutputMsgs"(w58) -> ()
        n400 = Array Size(array=w52) -> (size(s)=w51:i32)
        n401 = local read "toChanger"() -> (w48:T1)
        n402 = while {
          tunnel: w52 -> [w89] mode=indexing
          tunnel: w51 -> [w86]
          i -> [w87]
          stop <- w80 stop-if-true
          n403 = local read "End Number"() -> (w88:i32)
          n404 = Unbundle By Name(w89) -> ("MSG"=w85:i16)
          n405 = Equal?(x=w86, y=w87) -> (x = y?=w81:bool)
          n406 = Equal?(x=w85, y=i16 -1) -> (x = y?=w82:bool)
          n407 = Equal?(x=w85, y=w88) -> ()  [unwired: 1 out]
          n408 = case shown="False" FALSE {
            tunnel: [FALSE ("Верификация запущена") TRUE ("Верификация запущена")] -> w83
            frame False {
            }
            frame True {
              w91 = T8."Disabled and Grayed Out" ("Disabled")
              n409 = flat-sequence {
                frame #0 {
                  n410 = dll-call lib="C:/Users/Татьяна Лях/Downloads/MyComplex-master/DLL-s/MakeFullImmitationStepDLL/Release/MakeFullImmitationStepDLL.dll" fn="?freeAllDlls@@YAXXZ" label="FREE DLLs"() -> ()  [unwired: 4 in, 2 out]
                  n411 = local write "Верификация запущена"(FALSE ("Верификация запущена")) -> ()
                }
                frame #1 {
                  n412 = One Button Dialog(message="Верификация завершена!") -> ()  [unwired: 1 in, 1 out]
                }
              }
              n413 = property on="START Button" class="Bool (strict)"("DisabledEnum"=T8."Enabled" ("Disabled")) -> ()  [unwired: 2 in, 2 out]
              n414 = property on="Stop Ver Button" class="Bool (strict)"("DisabledEnum"=w91) -> ()  [unwired: 2 in, 2 out]
              n415 = property on="Pause" class="Bool (strict)"("DisabledEnum"=w91) -> ()  [unwired: 2 in, 2 out]
            }
          }
          n416 = Compound Arithmetic op=OR(w83, w82, w81) -> (w80:bool)
        }
        n417 = call "Changer.vi"("toChanger"=w48, "out"=w49, "in"=w50) -> ()
      }
    }
    "Автоматический режим работы" <- "Режим работы:"
  }
  n418 = local write "Scalar"(TRUE ("Scalar")) -> ()
  "Project" <- "" ("Название проекта")
